vi "TGA_Main.vi"() -> ()   [LabVIEW 2016]
doc: "TGA Data Logger\n\n19-Aug-2021 R. Gibson"
uses:
  TGA_Furnace_v230504.llb/Euro_Data_cluster.ctl
  TGA_Furnace_v230504.llb/Balance_Data_cluster.ctl
  TGA_Furnace_v230504.llb/Eurotherm_3504_FP.ctl
  TGA_Furnace_v230504.llb/Eurotherm_3200_Modbus_Writeable.ctl
  TGA_Furnace_v230504.llb/Euro_Cmd_cluster.ctl
  TGA_Furnace_v230504.llb/Adam_Data_cluster.ctl
  TGA_Furnace_v230504.llb/Balance_cmd_cluster.ctl
  TGA_Furnace_v230504.llb/LogInterval.ctl
  TGA_Furnace_v230504.llb/ChartWidth.ctl
  TGA_Furnace_v230504.llb/ADAM_models_enu.ctl
  TGA_Furnace_v230504.llb/Adam_ID_cluster.ctl
  TGA_Furnace_v230504.llb/MFC_ID_cluster.ctl
  TGA_Furnace_v230504.llb/MFCs_ID_cluster.ctl
  TGA_Furnace_v230504.llb/HW_Config_cluster.ctl
  TGA_Furnace_v230504.llb/Config_cluster.ctl
  TGA_Furnace_v230504.llb/Euro_Data_cluster2.ctl
  TGA_Furnace_v230504.llb/Euro_Cmd_cluster_2.ctl
  TGA_Furnace_v230504.llb/_array_numeric_54x22.ctl
  TGA_Furnace_v230504.llb/Purge_State_enum.ctl
panel:
  out "Elapsed Time (hh:mm:ss)":string="00:00:00" caption="Elapsed Time"
  out "Logging":bool
  out "Sample#":i32 caption="# Logged"
  in  "LogInterval":T1=1 caption="Logging Interval:" items=["1 second"=1, "2 seconds"=2, "5 seconds"=5, "10 seconds"=10, "20 seconds"=20, "30 seconds"=30, "1 minute"=60, "2 minutes"=120, "5 minutes"=300]
  in  "StopLog_btn":bool
  in  "StartLog_btn":bool caption="Logging"
  out "stopping":bool=TRUE
  in  "stop":bool
  in  "Tab Control":T2(tab)
  out "MFC com error":bool caption="MFC\ncom error"
  out "Flow_status_cluster":T3
  in  "start_red_btn":bool
  in  "stop_red_btn":bool
  in  "reset_alarm_btn":bool
  in  "Zero_Balance_btn":bool
  in  "Tare_Balance_btn":bool
  out "Units":string
  out "balance_nodata":bool caption="Balance"
  out "Balance":dbl=nan caption="Mass (-offset)" format="%.3f"
  in  "offset_btn":bool
  in  "Temp_SP_btn":bool
  out "eurotherm_nodata":bool caption="Balance"
  out "Eurotherm_3504":T4={"PV"=nan, "SP"=nan, "OP"=nan} {"OP" format="%.2f"}
  out "adam_nodata":bool caption="Balance"
  out "Sample Temperature":dbl(slide)=nan scale=500.0..1800.0
  in  "chart":bool=TRUE caption="update"
  out "Waveform Chart":cluster{"Mass":dbl, "PV":dbl, dbl}(graph)={"Mass"=nan, "PV"=nan, nan}
  out "Gas_Flows 2":cluster{"N2":dbl, "H2":dbl, "CO":dbl, "CO2":dbl}={"N2"=nan, "H2"=nan, "CO"=nan, "CO2"=nan} caption="Gas_Flows (l/min)" {"CO2" format="%.2f"; "CO" format="%.2f"; "H2" format="%.2f"; "N2" format="%.2f"}
  out "N2_Alarm_2":bool
  out "Purge_state_indicator":T5(ring)
  out "Remaining":i32=284 caption="Seconds\nRemaining"
  in  "Update Graph":enum32{"Run", "Pause"}(radio) caption="Update Graph:"
  in  "clear_graph":bool
  out "XY Graph":cluster{dbl[], dbl[]}[](graph)=[{[3763419058.1468678, 3763419058.6469655, 3763419059.146789, 3763419059.647493, 3763419060.147222, 3763419060.6469135, 3763419061.146755, 3763419061.6469765, 3763419062.147566, 3763419062.647289, 3763419063.146896, 3763419063.6474705, 3763419064.147414, 3763419064.647183, 3763419065.0177894, 3763419192.4616065, 3763419192.961169, 3763419193.460889, 3763419193.9610443, 3763419194.461545, 3763419194.961543, 3763419195.460842, 3763419195.961084, 3763419196.4610868, 3763419196.961397, 3763419197.460931, 3763419197.961339, 3763419198.4614997, 3763419198.9607635, 3763419199.4611425, 3763419199.961304, 3763419200.4615474, 3763419200.960755, 3763419201.4607697, 3763419201.960702, 3763419202.4607854, 3763419202.9606795, 3763419203.460756, 3763419203.961436, 3763419204.4613805, 3763419204.961012, 3763419205.460958, 3763419205.960548, 3763419206.460789, 3763419206.9607215, 3763419207.461002, 3763419207.9605246, 3763419208.4611497, 3763419208.961407, 3763419209.461351, 3763419209.961406, 3763419210.460696, 3763419210.960537, 3763419211.460704, 3763419211.9607377, 3763419212.461395, 3763419212.961053, 3763419213.4614058, 3763419213.960675, 3763419214.4606533, 3763419214.9608603, 3763419215.4614525, 3763419215.9606404, 3763419216.4609637, 3763419216.9607835, 3763419217.4605246, 3763419217.961069, 3763419218.4613957, 3763419218.96064, 3763419219.4604506, 3763419219.961275, 3763419220.4606957, 3763419220.96139, 3763419221.4610434, 3763419221.960963, 3763419222.460838, 3763419222.9611554, 3763419223.4610176, 3763419223.961055, 3763419224.461224, 3763419224.9612026, 3763419225.2077017], [nan, nan, nan, nan, nan, nan, nan, nan, nan, nan, nan, nan, nan, nan, nan, nan, nan, nan, nan, nan, nan, nan, nan, nan, nan, nan, nan, nan, nan, nan, nan, nan, nan, nan, nan, nan, nan, nan, nan, nan, nan, nan, nan, nan, nan, nan, nan, nan, nan, nan, nan, nan, nan, nan, nan, nan, nan, nan, nan, nan, nan, nan, nan, nan, nan, nan, nan, nan, nan, nan, nan, nan, nan, nan, nan, nan, nan, nan, nan, nan, nan, nan]}, {[3763419058.1468678, 3763419058.6469655, 3763419059.146789, 3763419059.647493, 3763419060.147222, 3763419060.6469135, 3763419061.146755, 3763419061.6469765, 3763419062.147566, 3763419062.647289, 3763419063.146896, 3763419063.6474705, 3763419064.147414, 3763419064.647183, 3763419065.0177894, 3763419192.4616065, 3763419192.961169, 3763419193.460889, 3763419193.9610443, 3763419194.461545, 3763419194.961543, 3763419195.460842, 3763419195.961084, 3763419196.4610868, 3763419196.961397, 3763419197.460931, 3763419197.961339, 3763419198.4614997, 3763419198.9607635, 3763419199.4611425, 3763419199.961304, 3763419200.4615474, 3763419200.960755, 3763419201.4607697, 3763419201.960702, 3763419202.4607854, 3763419202.9606795, 3763419203.460756, 3763419203.961436, 3763419204.4613805, 3763419204.961012, 3763419205.460958, 3763419205.960548, 3763419206.460789, 3763419206.9607215, 3763419207.461002, 3763419207.9605246, 3763419208.4611497, 3763419208.961407, 3763419209.461351, 3763419209.961406, 3763419210.460696, 3763419210.960537, 3763419211.460704, 3763419211.9607377, 3763419212.461395, 3763419212.961053, 3763419213.4614058, 3763419213.960675, 3763419214.4606533, 3763419214.9608603, 3763419215.4614525, 3763419215.9606404, 3763419216.4609637, 3763419216.9607835, 3763419217.4605246, 3763419217.961069, 3763419218.4613957, 3763419218.96064, 3763419219.4604506, 3763419219.961275, 3763419220.4606957, 3763419220.96139, 3763419221.4610434, 3763419221.960963, 3763419222.460838, 3763419222.9611554, 3763419223.4610176, 3763419223.961055, 3763419224.461224, 3763419224.9612026, 3763419225.2077017], [nan, nan, nan, nan, nan, nan, nan, nan, nan, nan, nan, nan, nan, nan, nan, nan, nan, nan, nan, nan, nan, nan, nan, nan, nan, nan, nan, nan, nan, nan, nan, nan, nan, nan, nan, nan, nan, nan, nan, nan, nan, nan, nan, nan, nan, nan, nan, nan, nan, nan, nan, nan, nan, nan, nan, nan, nan, nan, nan, nan, nan, nan, nan, nan, nan, nan, nan, nan, nan, nan, nan, nan, nan, nan, nan, nan, nan, nan, nan, nan, nan, nan]}, {[3763419058.1468678, 3763419058.6469655, 3763419059.146789, 3763419059.647493, 3763419060.147222, 3763419060.6469135, 3763419061.146755, 3763419061.6469765, 3763419062.147566, 3763419062.647289, 3763419063.146896, 3763419063.6474705, 3763419064.147414, 3763419064.647183, 3763419065.0177894, 3763419192.4616065, 3763419192.961169, 3763419193.460889, 3763419193.9610443, 3763419194.461545, 3763419194.961543, 3763419195.460842, 3763419195.961084, 3763419196.4610868, 3763419196.961397, 3763419197.460931, 3763419197.961339, 3763419198.4614997, 3763419198.9607635, 3763419199.4611425, 3763419199.961304, 3763419200.4615474, 3763419200.960755, 3763419201.4607697, 3763419201.960702, 3763419202.4607854, 3763419202.9606795, 3763419203.460756, 3763419203.961436, 3763419204.4613805, 3763419204.961012, 3763419205.460958, 3763419205.960548, 3763419206.460789, 3763419206.9607215, 3763419207.461002, 3763419207.9605246, 3763419208.4611497, 3763419208.961407, 3763419209.461351, 3763419209.961406, 3763419210.460696, 3763419210.960537, 3763419211.460704, 3763419211.9607377, 3763419212.461395, 3763419212.961053, 3763419213.4614058, 3763419213.960675, 3763419214.4606533, 3763419214.9608603, 3763419215.4614525, 3763419215.9606404, 3763419216.4609637, 3763419216.9607835, 3763419217.4605246, 3763419217.961069, 3763419218.4613957, 3763419218.96064, 3763419219.4604506, 3763419219.961275, 3763419220.4606957, 3763419220.96139, 3763419221.4610434, 3763419221.960963, 3763419222.460838, 3763419222.9611554, 3763419223.4610176, 3763419223.961055, 3763419224.461224, 3763419224.9612026, 3763419225.2077017], [nan, nan, nan, nan, nan, nan, nan, nan, nan, nan, nan, nan, nan, nan, nan, nan, nan, nan, nan, nan, nan, nan, nan, nan, nan, nan, nan, nan, nan, nan, nan, nan, nan, nan, nan, nan, nan, nan, nan, nan, nan, nan, nan, nan, nan, nan, nan, nan, nan, nan, nan, nan, nan, nan, nan, nan, nan, nan, nan, nan, nan, nan, nan, nan, nan, nan, nan, nan, nan, nan, nan, nan, nan, nan, nan, nan, nan, nan, nan, nan, nan, nan]}]
  in  "GraphWidth":T6=1 caption="Graph Width" items=["1 Minute", "5 Minutes", "10 Minutes", "30 Minutes", "1 Hour", "2 Hours"]
  out "Cluster":T7={"Balance"=nan, "Furnace"=nan, "Sample"=nan} {"Balance" format="%.3f"}
  in  "test flow":dbl[](array[numeric])
  in  "Gas_Times":cluster{"Reduction Time":i32, "Purge Time":i32}={"Reduction Time"=600, "Purge Time"=300} caption="Gas Times"
  in  "Purge Flow":dbl=10.0 min=0.0 max=20.0
  in  "reset_btn2":bool
  out "N2_Alarm":bool caption="N2 Low Flow\nAlarm"
  in  "AlarmDelay":dbl=30.0 caption="N2 Low Flow\nAlarm Delay" min=1.0 max=600.0 step=1.0
  out "Gasfile_changed":bool
  out "Actual Flow (l/min)":dbl=nan caption="Total Flow" format="%.2f"
  out "Gas_Filename":string="Default+H" caption="Gas File Name"
  in  "gasfile_open_btn":bool
  in  "gasfile_saveas_btn":bool
  in  "gasfile_save_btn":bool
  in  "Gas_Controls":T8 caption="Gas On/off\nControls"
  in  "Gas Setpoints":T9={"Flow SP (l/min)"=15.0, "F1 N2 (%)"=68.0, "F1 H2 (%)"=2.0000000000000004, "F1 CO (%)"=10.0, "F1 CO2 (%)"=20.0} {"F1 H2 (%)" min=0.0 max=100.0 step=0.1 format="%.1f"; "F1 CO2 (%)" min=0.0 max=100.0 step=0.1 format="%.1f"; "F1 CO (%)" min=0.0 max=100.0 step=0.1 format="%.1f"; "F1 N2 (%)" min=-10.0 max=100.0 format="%.1f"; "Flow SP (l/min)" min=0.0 max=30.0 format="%.1f"}
  out "Sol Valve States":bool[](array[boolean])=[FALSE, FALSE, TRUE, TRUE] caption="MFC Solenoid \nValve State"
  out "MFC Loop (ms)":u32=913
  out "MFC Update":bool[](array[boolean]) caption="Update"
  out "Actual Flows (l/min)":T10[](array[typedef])=[nan, nan, nan, nan] caption="Actual\nFlows (l/min)" format="%.2f"
  out "Read Setpoints":T10[](array[typedef]) caption="Readback\nSetpoints" format="%.2f"
  out "MFC Errors":bool[](array[boolean])=[TRUE, TRUE, TRUE, TRUE] caption="Com\nError"
  out "MFC Scan":i32=4
  out "MFC Init. Error":bool[](array[boolean])=[TRUE, TRUE, TRUE, TRUE] caption="Init. \nError"
  out "TGA_select_valve":bool caption="TGA Select\nValve status"
  out "Gas_Flows":cluster{"N2":dbl, "H2":dbl, "CO":dbl, "CO2":dbl}={"N2"=nan, "H2"=nan, "CO"=nan, "CO2"=nan} caption="Gas_Flows\n(l/min)" {"CO2" format="%.2f"; "CO" format="%.2f"; "H2" format="%.2f"; "N2" format="%.2f"}
  in  "Flow_error%":dbl=20.0 caption="Low Flowrate\nDetect Error%" format="%#_13g"
  out "N2_Flow_state":u16(ring) caption="N2 Flow state"
  out "Purge_State":T11 caption="Gas State"
  in  "Purge Setpoints":T12={"F1 N2 (%)"=99.0, "F1 H2 (%)"=1.0, "F1 CO (%)"=0.0, "F1 CO2 (%)"=0.0} caption="Post-Purge Mix" {"F1 N2 (%)" format="%.1f"; "F1 CO (%)" min=0.0 max=10.0 format="%.1f"; "F1 CO2 (%)" min=0.0 max=50.0 format="%.1f"; "F1 H2 (%)" min=0.0 max=4.0 format="%.1f"}
  out "PrePurge Time":i32=300 caption="Pre-Reduction\nPurge Time"
  out "All Gas Off":bool=TRUE
  in  "Adam_Out_FB":u16=65280
  in  "Gas_SPs_Loaded":T9={"Flow SP (l/min)"=15.0, "F1 N2 (%)"=68.0, "F1 H2 (%)"=2.0000000000000004, "F1 CO (%)"=10.0, "F1 CO2 (%)"=20.0} {"F1 H2 (%)" min=0.0 max=100.0 step=0.1 format="%.1f"; "F1 CO2 (%)" min=0.0 max=100.0 step=0.1 format="%.1f"; "F1 CO (%)" min=0.0 max=100.0 step=0.1 format="%.1f"; "F1 N2 (%)" min=-10.0 max=100.0 format="%.1f"; "Flow SP (l/min)" min=0.0 max=30.0 format="%.1f"}
  out "cancel_purge":bool
  out "lock door":bool
  out "TGA_Gas_select":bool
  out "F2_Solenoid_On":bool
  out "F1_Solenoid_On":bool
  out "Adam_Out_Error":bool=TRUE
  out "Mass-Offset":dbl=nan caption="Mass-offset" format="%.4f"
  in  "LogEndComment":bool caption="Prompt for comment at end of logging"
  in  "LogStartComment":bool caption="Prompt for comment at start of logging."
  out "Filename":string
  in  "Data directory path":path=path "C:/TGA/Data"
  out "LogDivider":i32=1
  out "Mass":dbl=nan caption="Mass (g)" format="%.4f"
  in  "Mass_offset":dbl caption="Mass Offset" format="%.4f"
  in  "GraphSizeLimit":i32=7200 caption="Graph Size Limit (s)" min=300 max=86400
  out "ClearGraph":bool
  out "Log File Path":path
  out "ChrtWidth (s)":i32=300 caption="Graph Width (s)"
  out "Balance_Data_cluster":T13={"Cmd"="Error", "Stable"=FALSE, "Mass"=nan, "Units"=""}
  out "Euro_Data_cluster":T14={"Timestamp"=3763419225.2077017, "PV"=nan, "tSP"=nan, "T_OP"=nan, "wOP"=nan, "wSP"=nan} {"Timestamp" format="%<%I:%M:%S %p>T"; "wOP" format="%.1f"; "T_OP" format="%.1f"}
  out "Adam_Data_cluster":cluster{"ComError":bool, "Adam_Data":dbl[]}={"ComError"=TRUE, "Adam_Data"=[nan, nan, nan, nan, nan, nan, nan, nan]} caption="Adam_In_Data_cluster"
  out "MFCs Listbox":i32(listbox) caption="MFC IDs list"
  out "Config_Load_Error":bool caption="Config. File Load Error  -  Default values have been used."
  out "Config_Path":path=path "C:/TGA/TGA_Main_v230404.cfg" caption="Config Path:"
  out "HW_Config_display":T15={"Balance_Port"="COM4", "Adam_Input_Port"="COM6", "Euro_Port"="COM5", "Adam_Output_Port"="COM7", "MFCs_Port"="COM10"}
  out "Slide":u8(slide)=61
  out "Author:":string="Ross Gibson"
  out "Title:":string="TGA Furnace Data Logger"
  out "App Path:":string="C:\\Users\\rkg415\\Documents\\Projects\\NIER Projects\\TGA Furnace\\Software LV2016\\V230404"
  out "LabVIEW Version:":string="2016"
  out "Date:":string="19-Apr-2023"
  out "Version:":string="v230404"
  out "Program:":string="TGA_Main.vi"
  in  "Euro_cmd_Write Cluster":T17={"Value"=FALSE, "Writeable_Registers"=5225, "Writeable_Registers 2"=5227, "Value 2"=FALSE, "Writeable_Registers 3"=5226, "Value 3"=FALSE, "d/min"=5, "Writeable_Registers 4"=5381, "Writeable_Registers 5"=5382, "deg"=200, "Writeable_Registers 6"=5412, "(m)"=20, "Writeable_Registers 7"=5445, "d/min"=5, "Writeable_Registers 8"=5446, "deg"=20, "Writeable_Registers 9"=470, "Value 4"=FALSE} {"Writeable_Registers 9" items=["Autotune"=470, "P1_Seg3_TargetSP"=5446, "P1_Seg3_RampRate"=5445, "P1_Seg2_Duration"=5412, "P1_Seg1_TargetSP"=5382, "P1_Seg1_RampRate"=5381, "P1_Reset"=5225, "P1_Hold"=5227, "P1_Run"=5226, "TG.SP"=2, "MAN.OP"=3, "PB"=6, "CTRL.A"=7, "Ti"=8, "Td"=9, "RNG.LO"=11, "RNG.HI"=12, "A1.---"=13, "A2.---"=14, "SP.SEL"=15, "D.BAND"=16, "CB.Lo"=17, "CB.HI"=18, "R2G"=19, "MTR.T"=21, "T.STAT"=23, "SP1"=24, "SP2"=25, "Rm.SP"=26, "LOC.t"=27, "MR"=28, "OP.HI"=30, "OP.LO"=31, "SAFE"=34, "SP.RAT"=35, "A1.HYS"=47, "A2.HYS"=68, "A3.HYS"=69, "A4.HYS"=71, "LD.AMP"=80, "A3.---"=81, "A4.---"=82, "LBT"=83, "F.OP"=84, "F.MOD"=85, "HYST.H"=86, "HYST.C"=88, "FILT.T"=101, "RC.FT"=102, "RC.PV"=103, "Home"=106, "SP.HI"=111, "SP.LO"=112, "ADDR"=131, "PV.Offset"=141, "C.Adj"=146, "IM"=199, "MV.IN"=202, "PV.CM"=203, "SBR"=258, "NEW.AL"=260, "LBR"=263, "A.TUNE"=270, "A-M"=273, "Ac-All"=274, "L-R"=276, "REM.%"=277, "REM.HI"=278, "REM.LO"=279, "ROP.HI"=280, "ROP.LO"=281, "A1.STS"=294, "A2.STS"=295, "A3.STS"=296, "A4.STS"=297, "LD.ALM"=304, "LK.ALM"=305, "HC.ALM"=306, "LOAD.A"=307, "HILC.A"=309, "REC.NO"=313, "StOrE"=314, "TM.CFG"=320, "TM.RES"=321, "SS.SP"=322, "SS.PWR"=323, "DWELL"=324, "THRES"=327, "End.T"=328, "SERVO"=329, "EVENT"=331, "P.CYCL"=332, "CYCLE"=33, "CTRL.H"=512, "CTRL.C"=513, "PB.UNT"=514, "Lev2.P"=515, "UNITS"=516, "Lev3.P"=517, "Conf.P"=518, "Cold"=519, "PASS.C"=520, "PASS.2"=521, "COOL.t"=524, "DEC.P"=525, "STBY.T"=530, "RAMP.UNITS"=531, "Meter"=532, "uCAL"=533, "A1.TYP"=536, "A2.TYP"=537, "A3.TYP"=538, "A4.TYP"=539, "A1.LAT"=540, "A2.LAT"=541, "A3.LAT"=542, "A4.LAT"=543, "A1.BLK"=544, "A2.BLK"=545, "A3.BLK"=546, "A4.BLK"=547, "OFS.HI"=560, "OFS.LO"=561, "PNT.HI"=562, "PNT.LO"=563, "CT.RNG"=572, "Sb.tyP"=578, "Id"=629, "GO"=769, "AO.Cal"=775, "K.LOC"=1104, "Dwel.1"=1280, "TSP.1"=1281, "RMP.1"=1282, "Dwel.2"=1283, "TSP.2"=1284, "RMP.2"=1285, "Dwel.3"=1286, "TSP.3"=1287, "RMP.3"=1288, "Dwel.4"=1289, "TSP.4"=1290, "RMP.4"=1291, "AT.R2G"=4176, "IN.TYP"=12290, "CJ.tyP"=12291, "mV.HI"=12306, "mV.LO"=12307, "L.TYPE"=12352, "L.D.IN"=12353, "L.SENS"=12361, "L.TYPE (LB)"=12368, "L.D.IN (LB)"=12369, "L.SENS (LB)"=12377, "BAUD"=12548, "PRTY"=12549, "DELAY"=12550, "RETRN"=12551, "REG.AD"=12552, "Ct.Id"=12608, "CT.SRC"=12609, "CT.LAT"=12610, "1.D.IN"=12673, "1.Func"=12675, "1.RNG"=12676, "1.SRC.A"=12678, "1.SRC.B"=12679, "1.SRC.C"=12680, "1.SRC.D"=12681, "1.SENS"=12682, "1.PLS"=12706, "2.FUNC"=12739, "2.RNG"=12740, "2.SRC.A"=12742, "2.SRC.B"=12743, "2.SRC.C"=12744, "2.SRC.D"=12745, "2.SENS"=12746, "2.PLS"=12770, "3.FUNC"=12803, "3.RNG"=12804, "3.SRC.A"=12806, "3.SRC.B"=12807, "3.SRC.C"=12808, "3.SRC.D"=12809, "3.SENS"=12810, "3.PLS"=12834, "4.FUNC"=13059, "4.SRC.A"=13062, "4.SRC.B"=13063, "4.SRC.C"=13064, "4.SRC.D"=13065, "4.SENS"=13066, "4.PLS"=13090]; "Writeable_Registers 8" items=["Autotune"=470, "P1_Seg3_TargetSP"=5446, "P1_Seg3_RampRate"=5445, "P1_Seg2_Duration"=5412, "P1_Seg1_TargetSP"=5382, "P1_Seg1_RampRate"=5381, "P1_Reset"=5225, "P1_Hold"=5227, "P1_Run"=5226, "TG.SP"=2, "MAN.OP"=3, "PB"=6, "CTRL.A"=7, "Ti"=8, "Td"=9, "RNG.LO"=11, "RNG.HI"=12, "A1.---"=13, "A2.---"=14, "SP.SEL"=15, "D.BAND"=16, "CB.Lo"=17, "CB.HI"=18, "R2G"=19, "MTR.T"=21, "T.STAT"=23, "SP1"=24, "SP2"=25, "Rm.SP"=26, "LOC.t"=27, "MR"=28, "OP.HI"=30, "OP.LO"=31, "SAFE"=34, "SP.RAT"=35, "A1.HYS"=47, "A2.HYS"=68, "A3.HYS"=69, "A4.HYS"=71, "LD.AMP"=80, "A3.---"=81, "A4.---"=82, "LBT"=83, "F.OP"=84, "F.MOD"=85, "HYST.H"=86, "HYST.C"=88, "FILT.T"=101, "RC.FT"=102, "RC.PV"=103, "Home"=106, "SP.HI"=111, "SP.LO"=112, "ADDR"=131, "PV.Offset"=141, "C.Adj"=146, "IM"=199, "MV.IN"=202, "PV.CM"=203, "SBR"=258, "NEW.AL"=260, "LBR"=263, "A.TUNE"=270, "A-M"=273, "Ac-All"=274, "L-R"=276, "REM.%"=277, "REM.HI"=278, "REM.LO"=279, "ROP.HI"=280, "ROP.LO"=281, "A1.STS"=294, "A2.STS"=295, "A3.STS"=296, "A4.STS"=297, "LD.ALM"=304, "LK.ALM"=305, "HC.ALM"=306, "LOAD.A"=307, "HILC.A"=309, "REC.NO"=313, "StOrE"=314, "TM.CFG"=320, "TM.RES"=321, "SS.SP"=322, "SS.PWR"=323, "DWELL"=324, "THRES"=327, "End.T"=328, "SERVO"=329, "EVENT"=331, "P.CYCL"=332, "CYCLE"=33, "CTRL.H"=512, "CTRL.C"=513, "PB.UNT"=514, "Lev2.P"=515, "UNITS"=516, "Lev3.P"=517, "Conf.P"=518, "Cold"=519, "PASS.C"=520, "PASS.2"=521, "COOL.t"=524, "DEC.P"=525, "STBY.T"=530, "RAMP.UNITS"=531, "Meter"=532, "uCAL"=533, "A1.TYP"=536, "A2.TYP"=537, "A3.TYP"=538, "A4.TYP"=539, "A1.LAT"=540, "A2.LAT"=541, "A3.LAT"=542, "A4.LAT"=543, "A1.BLK"=544, "A2.BLK"=545, "A3.BLK"=546, "A4.BLK"=547, "OFS.HI"=560, "OFS.LO"=561, "PNT.HI"=562, "PNT.LO"=563, "CT.RNG"=572, "Sb.tyP"=578, "Id"=629, "GO"=769, "AO.Cal"=775, "K.LOC"=1104, "Dwel.1"=1280, "TSP.1"=1281, "RMP.1"=1282, "Dwel.2"=1283, "TSP.2"=1284, "RMP.2"=1285, "Dwel.3"=1286, "TSP.3"=1287, "RMP.3"=1288, "Dwel.4"=1289, "TSP.4"=1290, "RMP.4"=1291, "AT.R2G"=4176, "IN.TYP"=12290, "CJ.tyP"=12291, "mV.HI"=12306, "mV.LO"=12307, "L.TYPE"=12352, "L.D.IN"=12353, "L.SENS"=12361, "L.TYPE (LB)"=12368, "L.D.IN (LB)"=12369, "L.SENS (LB)"=12377, "BAUD"=12548, "PRTY"=12549, "DELAY"=12550, "RETRN"=12551, "REG.AD"=12552, "Ct.Id"=12608, "CT.SRC"=12609, "CT.LAT"=12610, "1.D.IN"=12673, "1.Func"=12675, "1.RNG"=12676, "1.SRC.A"=12678, "1.SRC.B"=12679, "1.SRC.C"=12680, "1.SRC.D"=12681, "1.SENS"=12682, "1.PLS"=12706, "2.FUNC"=12739, "2.RNG"=12740, "2.SRC.A"=12742, "2.SRC.B"=12743, "2.SRC.C"=12744, "2.SRC.D"=12745, "2.SENS"=12746, "2.PLS"=12770, "3.FUNC"=12803, "3.RNG"=12804, "3.SRC.A"=12806, "3.SRC.B"=12807, "3.SRC.C"=12808, "3.SRC.D"=12809, "3.SENS"=12810, "3.PLS"=12834, "4.FUNC"=13059, "4.SRC.A"=13062, "4.SRC.B"=13063, "4.SRC.C"=13064, "4.SRC.D"=13065, "4.SENS"=13066, "4.PLS"=13090]; "Writeable_Registers 7" items=["Autotune"=470, "P1_Seg3_TargetSP"=5446, "P1_Seg3_RampRate"=5445, "P1_Seg2_Duration"=5412, "P1_Seg1_TargetSP"=5382, "P1_Seg1_RampRate"=5381, "P1_Reset"=5225, "P1_Hold"=5227, "P1_Run"=5226, "TG.SP"=2, "MAN.OP"=3, "PB"=6, "CTRL.A"=7, "Ti"=8, "Td"=9, "RNG.LO"=11, "RNG.HI"=12, "A1.---"=13, "A2.---"=14, "SP.SEL"=15, "D.BAND"=16, "CB.Lo"=17, "CB.HI"=18, "R2G"=19, "MTR.T"=21, "T.STAT"=23, "SP1"=24, "SP2"=25, "Rm.SP"=26, "LOC.t"=27, "MR"=28, "OP.HI"=30, "OP.LO"=31, "SAFE"=34, "SP.RAT"=35, "A1.HYS"=47, "A2.HYS"=68, "A3.HYS"=69, "A4.HYS"=71, "LD.AMP"=80, "A3.---"=81, "A4.---"=82, "LBT"=83, "F.OP"=84, "F.MOD"=85, "HYST.H"=86, "HYST.C"=88, "FILT.T"=101, "RC.FT"=102, "RC.PV"=103, "Home"=106, "SP.HI"=111, "SP.LO"=112, "ADDR"=131, "PV.Offset"=141, "C.Adj"=146, "IM"=199, "MV.IN"=202, "PV.CM"=203, "SBR"=258, "NEW.AL"=260, "LBR"=263, "A.TUNE"=270, "A-M"=273, "Ac-All"=274, "L-R"=276, "REM.%"=277, "REM.HI"=278, "REM.LO"=279, "ROP.HI"=280, "ROP.LO"=281, "A1.STS"=294, "A2.STS"=295, "A3.STS"=296, "A4.STS"=297, "LD.ALM"=304, "LK.ALM"=305, "HC.ALM"=306, "LOAD.A"=307, "HILC.A"=309, "REC.NO"=313, "StOrE"=314, "TM.CFG"=320, "TM.RES"=321, "SS.SP"=322, "SS.PWR"=323, "DWELL"=324, "THRES"=327, "End.T"=328, "SERVO"=329, "EVENT"=331, "P.CYCL"=332, "CYCLE"=33, "CTRL.H"=512, "CTRL.C"=513, "PB.UNT"=514, "Lev2.P"=515, "UNITS"=516, "Lev3.P"=517, "Conf.P"=518, "Cold"=519, "PASS.C"=520, "PASS.2"=521, "COOL.t"=524, "DEC.P"=525, "STBY.T"=530, "RAMP.UNITS"=531, "Meter"=532, "uCAL"=533, "A1.TYP"=536, "A2.TYP"=537, "A3.TYP"=538, "A4.TYP"=539, "A1.LAT"=540, "A2.LAT"=541, "A3.LAT"=542, "A4.LAT"=543, "A1.BLK"=544, "A2.BLK"=545, "A3.BLK"=546, "A4.BLK"=547, "OFS.HI"=560, "OFS.LO"=561, "PNT.HI"=562, "PNT.LO"=563, "CT.RNG"=572, "Sb.tyP"=578, "Id"=629, "GO"=769, "AO.Cal"=775, "K.LOC"=1104, "Dwel.1"=1280, "TSP.1"=1281, "RMP.1"=1282, "Dwel.2"=1283, "TSP.2"=1284, "RMP.2"=1285, "Dwel.3"=1286, "TSP.3"=1287, "RMP.3"=1288, "Dwel.4"=1289, "TSP.4"=1290, "RMP.4"=1291, "AT.R2G"=4176, "IN.TYP"=12290, "CJ.tyP"=12291, "mV.HI"=12306, "mV.LO"=12307, "L.TYPE"=12352, "L.D.IN"=12353, "L.SENS"=12361, "L.TYPE (LB)"=12368, "L.D.IN (LB)"=12369, "L.SENS (LB)"=12377, "BAUD"=12548, "PRTY"=12549, "DELAY"=12550, "RETRN"=12551, "REG.AD"=12552, "Ct.Id"=12608, "CT.SRC"=12609, "CT.LAT"=12610, "1.D.IN"=12673, "1.Func"=12675, "1.RNG"=12676, "1.SRC.A"=12678, "1.SRC.B"=12679, "1.SRC.C"=12680, "1.SRC.D"=12681, "1.SENS"=12682, "1.PLS"=12706, "2.FUNC"=12739, "2.RNG"=12740, "2.SRC.A"=12742, "2.SRC.B"=12743, "2.SRC.C"=12744, "2.SRC.D"=12745, "2.SENS"=12746, "2.PLS"=12770, "3.FUNC"=12803, "3.RNG"=12804, "3.SRC.A"=12806, "3.SRC.B"=12807, "3.SRC.C"=12808, "3.SRC.D"=12809, "3.SENS"=12810, "3.PLS"=12834, "4.FUNC"=13059, "4.SRC.A"=13062, "4.SRC.B"=13063, "4.SRC.C"=13064, "4.SRC.D"=13065, "4.SENS"=13066, "4.PLS"=13090]; "Writeable_Registers 6" items=["Autotune"=470, "P1_Seg3_TargetSP"=5446, "P1_Seg3_RampRate"=5445, "P1_Seg2_Duration"=5412, "P1_Seg1_TargetSP"=5382, "P1_Seg1_RampRate"=5381, "P1_Reset"=5225, "P1_Hold"=5227, "P1_Run"=5226, "TG.SP"=2, "MAN.OP"=3, "PB"=6, "CTRL.A"=7, "Ti"=8, "Td"=9, "RNG.LO"=11, "RNG.HI"=12, "A1.---"=13, "A2.---"=14, "SP.SEL"=15, "D.BAND"=16, "CB.Lo"=17, "CB.HI"=18, "R2G"=19, "MTR.T"=21, "T.STAT"=23, "SP1"=24, "SP2"=25, "Rm.SP"=26, "LOC.t"=27, "MR"=28, "OP.HI"=30, "OP.LO"=31, "SAFE"=34, "SP.RAT"=35, "A1.HYS"=47, "A2.HYS"=68, "A3.HYS"=69, "A4.HYS"=71, "LD.AMP"=80, "A3.---"=81, "A4.---"=82, "LBT"=83, "F.OP"=84, "F.MOD"=85, "HYST.H"=86, "HYST.C"=88, "FILT.T"=101, "RC.FT"=102, "RC.PV"=103, "Home"=106, "SP.HI"=111, "SP.LO"=112, "ADDR"=131, "PV.Offset"=141, "C.Adj"=146, "IM"=199, "MV.IN"=202, "PV.CM"=203, "SBR"=258, "NEW.AL"=260, "LBR"=263, "A.TUNE"=270, "A-M"=273, "Ac-All"=274, "L-R"=276, "REM.%"=277, "REM.HI"=278, "REM.LO"=279, "ROP.HI"=280, "ROP.LO"=281, "A1.STS"=294, "A2.STS"=295, "A3.STS"=296, "A4.STS"=297, "LD.ALM"=304, "LK.ALM"=305, "HC.ALM"=306, "LOAD.A"=307, "HILC.A"=309, "REC.NO"=313, "StOrE"=314, "TM.CFG"=320, "TM.RES"=321, "SS.SP"=322, "SS.PWR"=323, "DWELL"=324, "THRES"=327, "End.T"=328, "SERVO"=329, "EVENT"=331, "P.CYCL"=332, "CYCLE"=33, "CTRL.H"=512, "CTRL.C"=513, "PB.UNT"=514, "Lev2.P"=515, "UNITS"=516, "Lev3.P"=517, "Conf.P"=518, "Cold"=519, "PASS.C"=520, "PASS.2"=521, "COOL.t"=524, "DEC.P"=525, "STBY.T"=530, "RAMP.UNITS"=531, "Meter"=532, "uCAL"=533, "A1.TYP"=536, "A2.TYP"=537, "A3.TYP"=538, "A4.TYP"=539, "A1.LAT"=540, "A2.LAT"=541, "A3.LAT"=542, "A4.LAT"=543, "A1.BLK"=544, "A2.BLK"=545, "A3.BLK"=546, "A4.BLK"=547, "OFS.HI"=560, "OFS.LO"=561, "PNT.HI"=562, "PNT.LO"=563, "CT.RNG"=572, "Sb.tyP"=578, "Id"=629, "GO"=769, "AO.Cal"=775, "K.LOC"=1104, "Dwel.1"=1280, "TSP.1"=1281, "RMP.1"=1282, "Dwel.2"=1283, "TSP.2"=1284, "RMP.2"=1285, "Dwel.3"=1286, "TSP.3"=1287, "RMP.3"=1288, "Dwel.4"=1289, "TSP.4"=1290, "RMP.4"=1291, "AT.R2G"=4176, "IN.TYP"=12290, "CJ.tyP"=12291, "mV.HI"=12306, "mV.LO"=12307, "L.TYPE"=12352, "L.D.IN"=12353, "L.SENS"=12361, "L.TYPE (LB)"=12368, "L.D.IN (LB)"=12369, "L.SENS (LB)"=12377, "BAUD"=12548, "PRTY"=12549, "DELAY"=12550, "RETRN"=12551, "REG.AD"=12552, "Ct.Id"=12608, "CT.SRC"=12609, "CT.LAT"=12610, "1.D.IN"=12673, "1.Func"=12675, "1.RNG"=12676, "1.SRC.A"=12678, "1.SRC.B"=12679, "1.SRC.C"=12680, "1.SRC.D"=12681, "1.SENS"=12682, "1.PLS"=12706, "2.FUNC"=12739, "2.RNG"=12740, "2.SRC.A"=12742, "2.SRC.B"=12743, "2.SRC.C"=12744, "2.SRC.D"=12745, "2.SENS"=12746, "2.PLS"=12770, "3.FUNC"=12803, "3.RNG"=12804, "3.SRC.A"=12806, "3.SRC.B"=12807, "3.SRC.C"=12808, "3.SRC.D"=12809, "3.SENS"=12810, "3.PLS"=12834, "4.FUNC"=13059, "4.SRC.A"=13062, "4.SRC.B"=13063, "4.SRC.C"=13064, "4.SRC.D"=13065, "4.SENS"=13066, "4.PLS"=13090]; "Writeable_Registers 5" items=["Autotune"=470, "P1_Seg3_TargetSP"=5446, "P1_Seg3_RampRate"=5445, "P1_Seg2_Duration"=5412, "P1_Seg1_TargetSP"=5382, "P1_Seg1_RampRate"=5381, "P1_Reset"=5225, "P1_Hold"=5227, "P1_Run"=5226, "TG.SP"=2, "MAN.OP"=3, "PB"=6, "CTRL.A"=7, "Ti"=8, "Td"=9, "RNG.LO"=11, "RNG.HI"=12, "A1.---"=13, "A2.---"=14, "SP.SEL"=15, "D.BAND"=16, "CB.Lo"=17, "CB.HI"=18, "R2G"=19, "MTR.T"=21, "T.STAT"=23, "SP1"=24, "SP2"=25, "Rm.SP"=26, "LOC.t"=27, "MR"=28, "OP.HI"=30, "OP.LO"=31, "SAFE"=34, "SP.RAT"=35, "A1.HYS"=47, "A2.HYS"=68, "A3.HYS"=69, "A4.HYS"=71, "LD.AMP"=80, "A3.---"=81, "A4.---"=82, "LBT"=83, "F.OP"=84, "F.MOD"=85, "HYST.H"=86, "HYST.C"=88, "FILT.T"=101, "RC.FT"=102, "RC.PV"=103, "Home"=106, "SP.HI"=111, "SP.LO"=112, "ADDR"=131, "PV.Offset"=141, "C.Adj"=146, "IM"=199, "MV.IN"=202, "PV.CM"=203, "SBR"=258, "NEW.AL"=260, "LBR"=263, "A.TUNE"=270, "A-M"=273, "Ac-All"=274, "L-R"=276, "REM.%"=277, "REM.HI"=278, "REM.LO"=279, "ROP.HI"=280, "ROP.LO"=281, "A1.STS"=294, "A2.STS"=295, "A3.STS"=296, "A4.STS"=297, "LD.ALM"=304, "LK.ALM"=305, "HC.ALM"=306, "LOAD.A"=307, "HILC.A"=309, "REC.NO"=313, "StOrE"=314, "TM.CFG"=320, "TM.RES"=321, "SS.SP"=322, "SS.PWR"=323, "DWELL"=324, "THRES"=327, "End.T"=328, "SERVO"=329, "EVENT"=331, "P.CYCL"=332, "CYCLE"=33, "CTRL.H"=512, "CTRL.C"=513, "PB.UNT"=514, "Lev2.P"=515, "UNITS"=516, "Lev3.P"=517, "Conf.P"=518, "Cold"=519, "PASS.C"=520, "PASS.2"=521, "COOL.t"=524, "DEC.P"=525, "STBY.T"=530, "RAMP.UNITS"=531, "Meter"=532, "uCAL"=533, "A1.TYP"=536, "A2.TYP"=537, "A3.TYP"=538, "A4.TYP"=539, "A1.LAT"=540, "A2.LAT"=541, "A3.LAT"=542, "A4.LAT"=543, "A1.BLK"=544, "A2.BLK"=545, "A3.BLK"=546, "A4.BLK"=547, "OFS.HI"=560, "OFS.LO"=561, "PNT.HI"=562, "PNT.LO"=563, "CT.RNG"=572, "Sb.tyP"=578, "Id"=629, "GO"=769, "AO.Cal"=775, "K.LOC"=1104, "Dwel.1"=1280, "TSP.1"=1281, "RMP.1"=1282, "Dwel.2"=1283, "TSP.2"=1284, "RMP.2"=1285, "Dwel.3"=1286, "TSP.3"=1287, "RMP.3"=1288, "Dwel.4"=1289, "TSP.4"=1290, "RMP.4"=1291, "AT.R2G"=4176, "IN.TYP"=12290, "CJ.tyP"=12291, "mV.HI"=12306, "mV.LO"=12307, "L.TYPE"=12352, "L.D.IN"=12353, "L.SENS"=12361, "L.TYPE (LB)"=12368, "L.D.IN (LB)"=12369, "L.SENS (LB)"=12377, "BAUD"=12548, "PRTY"=12549, "DELAY"=12550, "RETRN"=12551, "REG.AD"=12552, "Ct.Id"=12608, "CT.SRC"=12609, "CT.LAT"=12610, "1.D.IN"=12673, "1.Func"=12675, "1.RNG"=12676, "1.SRC.A"=12678, "1.SRC.B"=12679, "1.SRC.C"=12680, "1.SRC.D"=12681, "1.SENS"=12682, "1.PLS"=12706, "2.FUNC"=12739, "2.RNG"=12740, "2.SRC.A"=12742, "2.SRC.B"=12743, "2.SRC.C"=12744, "2.SRC.D"=12745, "2.SENS"=12746, "2.PLS"=12770, "3.FUNC"=12803, "3.RNG"=12804, "3.SRC.A"=12806, "3.SRC.B"=12807, "3.SRC.C"=12808, "3.SRC.D"=12809, "3.SENS"=12810, "3.PLS"=12834, "4.FUNC"=13059, "4.SRC.A"=13062, "4.SRC.B"=13063, "4.SRC.C"=13064, "4.SRC.D"=13065, "4.SENS"=13066, "4.PLS"=13090]; "Writeable_Registers 4" items=["Autotune"=470, "P1_Seg3_TargetSP"=5446, "P1_Seg3_RampRate"=5445, "P1_Seg2_Duration"=5412, "P1_Seg1_TargetSP"=5382, "P1_Seg1_RampRate"=5381, "P1_Reset"=5225, "P1_Hold"=5227, "P1_Run"=5226, "TG.SP"=2, "MAN.OP"=3, "PB"=6, "CTRL.A"=7, "Ti"=8, "Td"=9, "RNG.LO"=11, "RNG.HI"=12, "A1.---"=13, "A2.---"=14, "SP.SEL"=15, "D.BAND"=16, "CB.Lo"=17, "CB.HI"=18, "R2G"=19, "MTR.T"=21, "T.STAT"=23, "SP1"=24, "SP2"=25, "Rm.SP"=26, "LOC.t"=27, "MR"=28, "OP.HI"=30, "OP.LO"=31, "SAFE"=34, "SP.RAT"=35, "A1.HYS"=47, "A2.HYS"=68, "A3.HYS"=69, "A4.HYS"=71, "LD.AMP"=80, "A3.---"=81, "A4.---"=82, "LBT"=83, "F.OP"=84, "F.MOD"=85, "HYST.H"=86, "HYST.C"=88, "FILT.T"=101, "RC.FT"=102, "RC.PV"=103, "Home"=106, "SP.HI"=111, "SP.LO"=112, "ADDR"=131, "PV.Offset"=141, "C.Adj"=146, "IM"=199, "MV.IN"=202, "PV.CM"=203, "SBR"=258, "NEW.AL"=260, "LBR"=263, "A.TUNE"=270, "A-M"=273, "Ac-All"=274, "L-R"=276, "REM.%"=277, "REM.HI"=278, "REM.LO"=279, "ROP.HI"=280, "ROP.LO"=281, "A1.STS"=294, "A2.STS"=295, "A3.STS"=296, "A4.STS"=297, "LD.ALM"=304, "LK.ALM"=305, "HC.ALM"=306, "LOAD.A"=307, "HILC.A"=309, "REC.NO"=313, "StOrE"=314, "TM.CFG"=320, "TM.RES"=321, "SS.SP"=322, "SS.PWR"=323, "DWELL"=324, "THRES"=327, "End.T"=328, "SERVO"=329, "EVENT"=331, "P.CYCL"=332, "CYCLE"=33, "CTRL.H"=512, "CTRL.C"=513, "PB.UNT"=514, "Lev2.P"=515, "UNITS"=516, "Lev3.P"=517, "Conf.P"=518, "Cold"=519, "PASS.C"=520, "PASS.2"=521, "COOL.t"=524, "DEC.P"=525, "STBY.T"=530, "RAMP.UNITS"=531, "Meter"=532, "uCAL"=533, "A1.TYP"=536, "A2.TYP"=537, "A3.TYP"=538, "A4.TYP"=539, "A1.LAT"=540, "A2.LAT"=541, "A3.LAT"=542, "A4.LAT"=543, "A1.BLK"=544, "A2.BLK"=545, "A3.BLK"=546, "A4.BLK"=547, "OFS.HI"=560, "OFS.LO"=561, "PNT.HI"=562, "PNT.LO"=563, "CT.RNG"=572, "Sb.tyP"=578, "Id"=629, "GO"=769, "AO.Cal"=775, "K.LOC"=1104, "Dwel.1"=1280, "TSP.1"=1281, "RMP.1"=1282, "Dwel.2"=1283, "TSP.2"=1284, "RMP.2"=1285, "Dwel.3"=1286, "TSP.3"=1287, "RMP.3"=1288, "Dwel.4"=1289, "TSP.4"=1290, "RMP.4"=1291, "AT.R2G"=4176, "IN.TYP"=12290, "CJ.tyP"=12291, "mV.HI"=12306, "mV.LO"=12307, "L.TYPE"=12352, "L.D.IN"=12353, "L.SENS"=12361, "L.TYPE (LB)"=12368, "L.D.IN (LB)"=12369, "L.SENS (LB)"=12377, "BAUD"=12548, "PRTY"=12549, "DELAY"=12550, "RETRN"=12551, "REG.AD"=12552, "Ct.Id"=12608, "CT.SRC"=12609, "CT.LAT"=12610, "1.D.IN"=12673, "1.Func"=12675, "1.RNG"=12676, "1.SRC.A"=12678, "1.SRC.B"=12679, "1.SRC.C"=12680, "1.SRC.D"=12681, "1.SENS"=12682, "1.PLS"=12706, "2.FUNC"=12739, "2.RNG"=12740, "2.SRC.A"=12742, "2.SRC.B"=12743, "2.SRC.C"=12744, "2.SRC.D"=12745, "2.SENS"=12746, "2.PLS"=12770, "3.FUNC"=12803, "3.RNG"=12804, "3.SRC.A"=12806, "3.SRC.B"=12807, "3.SRC.C"=12808, "3.SRC.D"=12809, "3.SENS"=12810, "3.PLS"=12834, "4.FUNC"=13059, "4.SRC.A"=13062, "4.SRC.B"=13063, "4.SRC.C"=13064, "4.SRC.D"=13065, "4.SENS"=13066, "4.PLS"=13090]; "Writeable_Registers 3" items=["Autotune"=470, "P1_Seg3_TargetSP"=5446, "P1_Seg3_RampRate"=5445, "P1_Seg2_Duration"=5412, "P1_Seg1_TargetSP"=5382, "P1_Seg1_RampRate"=5381, "P1_Reset"=5225, "P1_Hold"=5227, "P1_Run"=5226, "TG.SP"=2, "MAN.OP"=3, "PB"=6, "CTRL.A"=7, "Ti"=8, "Td"=9, "RNG.LO"=11, "RNG.HI"=12, "A1.---"=13, "A2.---"=14, "SP.SEL"=15, "D.BAND"=16, "CB.Lo"=17, "CB.HI"=18, "R2G"=19, "MTR.T"=21, "T.STAT"=23, "SP1"=24, "SP2"=25, "Rm.SP"=26, "LOC.t"=27, "MR"=28, "OP.HI"=30, "OP.LO"=31, "SAFE"=34, "SP.RAT"=35, "A1.HYS"=47, "A2.HYS"=68, "A3.HYS"=69, "A4.HYS"=71, "LD.AMP"=80, "A3.---"=81, "A4.---"=82, "LBT"=83, "F.OP"=84, "F.MOD"=85, "HYST.H"=86, "HYST.C"=88, "FILT.T"=101, "RC.FT"=102, "RC.PV"=103, "Home"=106, "SP.HI"=111, "SP.LO"=112, "ADDR"=131, "PV.Offset"=141, "C.Adj"=146, "IM"=199, "MV.IN"=202, "PV.CM"=203, "SBR"=258, "NEW.AL"=260, "LBR"=263, "A.TUNE"=270, "A-M"=273, "Ac-All"=274, "L-R"=276, "REM.%"=277, "REM.HI"=278, "REM.LO"=279, "ROP.HI"=280, "ROP.LO"=281, "A1.STS"=294, "A2.STS"=295, "A3.STS"=296, "A4.STS"=297, "LD.ALM"=304, "LK.ALM"=305, "HC.ALM"=306, "LOAD.A"=307, "HILC.A"=309, "REC.NO"=313, "StOrE"=314, "TM.CFG"=320, "TM.RES"=321, "SS.SP"=322, "SS.PWR"=323, "DWELL"=324, "THRES"=327, "End.T"=328, "SERVO"=329, "EVENT"=331, "P.CYCL"=332, "CYCLE"=33, "CTRL.H"=512, "CTRL.C"=513, "PB.UNT"=514, "Lev2.P"=515, "UNITS"=516, "Lev3.P"=517, "Conf.P"=518, "Cold"=519, "PASS.C"=520, "PASS.2"=521, "COOL.t"=524, "DEC.P"=525, "STBY.T"=530, "RAMP.UNITS"=531, "Meter"=532, "uCAL"=533, "A1.TYP"=536, "A2.TYP"=537, "A3.TYP"=538, "A4.TYP"=539, "A1.LAT"=540, "A2.LAT"=541, "A3.LAT"=542, "A4.LAT"=543, "A1.BLK"=544, "A2.BLK"=545, "A3.BLK"=546, "A4.BLK"=547, "OFS.HI"=560, "OFS.LO"=561, "PNT.HI"=562, "PNT.LO"=563, "CT.RNG"=572, "Sb.tyP"=578, "Id"=629, "GO"=769, "AO.Cal"=775, "K.LOC"=1104, "Dwel.1"=1280, "TSP.1"=1281, "RMP.1"=1282, "Dwel.2"=1283, "TSP.2"=1284, "RMP.2"=1285, "Dwel.3"=1286, "TSP.3"=1287, "RMP.3"=1288, "Dwel.4"=1289, "TSP.4"=1290, "RMP.4"=1291, "AT.R2G"=4176, "IN.TYP"=12290, "CJ.tyP"=12291, "mV.HI"=12306, "mV.LO"=12307, "L.TYPE"=12352, "L.D.IN"=12353, "L.SENS"=12361, "L.TYPE (LB)"=12368, "L.D.IN (LB)"=12369, "L.SENS (LB)"=12377, "BAUD"=12548, "PRTY"=12549, "DELAY"=12550, "RETRN"=12551, "REG.AD"=12552, "Ct.Id"=12608, "CT.SRC"=12609, "CT.LAT"=12610, "1.D.IN"=12673, "1.Func"=12675, "1.RNG"=12676, "1.SRC.A"=12678, "1.SRC.B"=12679, "1.SRC.C"=12680, "1.SRC.D"=12681, "1.SENS"=12682, "1.PLS"=12706, "2.FUNC"=12739, "2.RNG"=12740, "2.SRC.A"=12742, "2.SRC.B"=12743, "2.SRC.C"=12744, "2.SRC.D"=12745, "2.SENS"=12746, "2.PLS"=12770, "3.FUNC"=12803, "3.RNG"=12804, "3.SRC.A"=12806, "3.SRC.B"=12807, "3.SRC.C"=12808, "3.SRC.D"=12809, "3.SENS"=12810, "3.PLS"=12834, "4.FUNC"=13059, "4.SRC.A"=13062, "4.SRC.B"=13063, "4.SRC.C"=13064, "4.SRC.D"=13065, "4.SENS"=13066, "4.PLS"=13090]; "Writeable_Registers 2" items=["Autotune"=470, "P1_Seg3_TargetSP"=5446, "P1_Seg3_RampRate"=5445, "P1_Seg2_Duration"=5412, "P1_Seg1_TargetSP"=5382, "P1_Seg1_RampRate"=5381, "P1_Reset"=5225, "P1_Hold"=5227, "P1_Run"=5226, "TG.SP"=2, "MAN.OP"=3, "PB"=6, "CTRL.A"=7, "Ti"=8, "Td"=9, "RNG.LO"=11, "RNG.HI"=12, "A1.---"=13, "A2.---"=14, "SP.SEL"=15, "D.BAND"=16, "CB.Lo"=17, "CB.HI"=18, "R2G"=19, "MTR.T"=21, "T.STAT"=23, "SP1"=24, "SP2"=25, "Rm.SP"=26, "LOC.t"=27, "MR"=28, "OP.HI"=30, "OP.LO"=31, "SAFE"=34, "SP.RAT"=35, "A1.HYS"=47, "A2.HYS"=68, "A3.HYS"=69, "A4.HYS"=71, "LD.AMP"=80, "A3.---"=81, "A4.---"=82, "LBT"=83, "F.OP"=84, "F.MOD"=85, "HYST.H"=86, "HYST.C"=88, "FILT.T"=101, "RC.FT"=102, "RC.PV"=103, "Home"=106, "SP.HI"=111, "SP.LO"=112, "ADDR"=131, "PV.Offset"=141, "C.Adj"=146, "IM"=199, "MV.IN"=202, "PV.CM"=203, "SBR"=258, "NEW.AL"=260, "LBR"=263, "A.TUNE"=270, "A-M"=273, "Ac-All"=274, "L-R"=276, "REM.%"=277, "REM.HI"=278, "REM.LO"=279, "ROP.HI"=280, "ROP.LO"=281, "A1.STS"=294, "A2.STS"=295, "A3.STS"=296, "A4.STS"=297, "LD.ALM"=304, "LK.ALM"=305, "HC.ALM"=306, "LOAD.A"=307, "HILC.A"=309, "REC.NO"=313, "StOrE"=314, "TM.CFG"=320, "TM.RES"=321, "SS.SP"=322, "SS.PWR"=323, "DWELL"=324, "THRES"=327, "End.T"=328, "SERVO"=329, "EVENT"=331, "P.CYCL"=332, "CYCLE"=33, "CTRL.H"=512, "CTRL.C"=513, "PB.UNT"=514, "Lev2.P"=515, "UNITS"=516, "Lev3.P"=517, "Conf.P"=518, "Cold"=519, "PASS.C"=520, "PASS.2"=521, "COOL.t"=524, "DEC.P"=525, "STBY.T"=530, "RAMP.UNITS"=531, "Meter"=532, "uCAL"=533, "A1.TYP"=536, "A2.TYP"=537, "A3.TYP"=538, "A4.TYP"=539, "A1.LAT"=540, "A2.LAT"=541, "A3.LAT"=542, "A4.LAT"=543, "A1.BLK"=544, "A2.BLK"=545, "A3.BLK"=546, "A4.BLK"=547, "OFS.HI"=560, "OFS.LO"=561, "PNT.HI"=562, "PNT.LO"=563, "CT.RNG"=572, "Sb.tyP"=578, "Id"=629, "GO"=769, "AO.Cal"=775, "K.LOC"=1104, "Dwel.1"=1280, "TSP.1"=1281, "RMP.1"=1282, "Dwel.2"=1283, "TSP.2"=1284, "RMP.2"=1285, "Dwel.3"=1286, "TSP.3"=1287, "RMP.3"=1288, "Dwel.4"=1289, "TSP.4"=1290, "RMP.4"=1291, "AT.R2G"=4176, "IN.TYP"=12290, "CJ.tyP"=12291, "mV.HI"=12306, "mV.LO"=12307, "L.TYPE"=12352, "L.D.IN"=12353, "L.SENS"=12361, "L.TYPE (LB)"=12368, "L.D.IN (LB)"=12369, "L.SENS (LB)"=12377, "BAUD"=12548, "PRTY"=12549, "DELAY"=12550, "RETRN"=12551, "REG.AD"=12552, "Ct.Id"=12608, "CT.SRC"=12609, "CT.LAT"=12610, "1.D.IN"=12673, "1.Func"=12675, "1.RNG"=12676, "1.SRC.A"=12678, "1.SRC.B"=12679, "1.SRC.C"=12680, "1.SRC.D"=12681, "1.SENS"=12682, "1.PLS"=12706, "2.FUNC"=12739, "2.RNG"=12740, "2.SRC.A"=12742, "2.SRC.B"=12743, "2.SRC.C"=12744, "2.SRC.D"=12745, "2.SENS"=12746, "2.PLS"=12770, "3.FUNC"=12803, "3.RNG"=12804, "3.SRC.A"=12806, "3.SRC.B"=12807, "3.SRC.C"=12808, "3.SRC.D"=12809, "3.SENS"=12810, "3.PLS"=12834, "4.FUNC"=13059, "4.SRC.A"=13062, "4.SRC.B"=13063, "4.SRC.C"=13064, "4.SRC.D"=13065, "4.SENS"=13066, "4.PLS"=13090]; "Writeable_Registers" items=["Autotune"=470, "P1_Seg3_TargetSP"=5446, "P1_Seg3_RampRate"=5445, "P1_Seg2_Duration"=5412, "P1_Seg1_TargetSP"=5382, "P1_Seg1_RampRate"=5381, "P1_Reset"=5225, "P1_Hold"=5227, "P1_Run"=5226, "TG.SP"=2, "MAN.OP"=3, "PB"=6, "CTRL.A"=7, "Ti"=8, "Td"=9, "RNG.LO"=11, "RNG.HI"=12, "A1.---"=13, "A2.---"=14, "SP.SEL"=15, "D.BAND"=16, "CB.Lo"=17, "CB.HI"=18, "R2G"=19, "MTR.T"=21, "T.STAT"=23, "SP1"=24, "SP2"=25, "Rm.SP"=26, "LOC.t"=27, "MR"=28, "OP.HI"=30, "OP.LO"=31, "SAFE"=34, "SP.RAT"=35, "A1.HYS"=47, "A2.HYS"=68, "A3.HYS"=69, "A4.HYS"=71, "LD.AMP"=80, "A3.---"=81, "A4.---"=82, "LBT"=83, "F.OP"=84, "F.MOD"=85, "HYST.H"=86, "HYST.C"=88, "FILT.T"=101, "RC.FT"=102, "RC.PV"=103, "Home"=106, "SP.HI"=111, "SP.LO"=112, "ADDR"=131, "PV.Offset"=141, "C.Adj"=146, "IM"=199, "MV.IN"=202, "PV.CM"=203, "SBR"=258, "NEW.AL"=260, "LBR"=263, "A.TUNE"=270, "A-M"=273, "Ac-All"=274, "L-R"=276, "REM.%"=277, "REM.HI"=278, "REM.LO"=279, "ROP.HI"=280, "ROP.LO"=281, "A1.STS"=294, "A2.STS"=295, "A3.STS"=296, "A4.STS"=297, "LD.ALM"=304, "LK.ALM"=305, "HC.ALM"=306, "LOAD.A"=307, "HILC.A"=309, "REC.NO"=313, "StOrE"=314, "TM.CFG"=320, "TM.RES"=321, "SS.SP"=322, "SS.PWR"=323, "DWELL"=324, "THRES"=327, "End.T"=328, "SERVO"=329, "EVENT"=331, "P.CYCL"=332, "CYCLE"=33, "CTRL.H"=512, "CTRL.C"=513, "PB.UNT"=514, "Lev2.P"=515, "UNITS"=516, "Lev3.P"=517, "Conf.P"=518, "Cold"=519, "PASS.C"=520, "PASS.2"=521, "COOL.t"=524, "DEC.P"=525, "STBY.T"=530, "RAMP.UNITS"=531, "Meter"=532, "uCAL"=533, "A1.TYP"=536, "A2.TYP"=537, "A3.TYP"=538, "A4.TYP"=539, "A1.LAT"=540, "A2.LAT"=541, "A3.LAT"=542, "A4.LAT"=543, "A1.BLK"=544, "A2.BLK"=545, "A3.BLK"=546, "A4.BLK"=547, "OFS.HI"=560, "OFS.LO"=561, "PNT.HI"=562, "PNT.LO"=563, "CT.RNG"=572, "Sb.tyP"=578, "Id"=629, "GO"=769, "AO.Cal"=775, "K.LOC"=1104, "Dwel.1"=1280, "TSP.1"=1281, "RMP.1"=1282, "Dwel.2"=1283, "TSP.2"=1284, "RMP.2"=1285, "Dwel.3"=1286, "TSP.3"=1287, "RMP.3"=1288, "Dwel.4"=1289, "TSP.4"=1290, "RMP.4"=1291, "AT.R2G"=4176, "IN.TYP"=12290, "CJ.tyP"=12291, "mV.HI"=12306, "mV.LO"=12307, "L.TYPE"=12352, "L.D.IN"=12353, "L.SENS"=12361, "L.TYPE (LB)"=12368, "L.D.IN (LB)"=12369, "L.SENS (LB)"=12377, "BAUD"=12548, "PRTY"=12549, "DELAY"=12550, "RETRN"=12551, "REG.AD"=12552, "Ct.Id"=12608, "CT.SRC"=12609, "CT.LAT"=12610, "1.D.IN"=12673, "1.Func"=12675, "1.RNG"=12676, "1.SRC.A"=12678, "1.SRC.B"=12679, "1.SRC.C"=12680, "1.SRC.D"=12681, "1.SENS"=12682, "1.PLS"=12706, "2.FUNC"=12739, "2.RNG"=12740, "2.SRC.A"=12742, "2.SRC.B"=12743, "2.SRC.C"=12744, "2.SRC.D"=12745, "2.SENS"=12746, "2.PLS"=12770, "3.FUNC"=12803, "3.RNG"=12804, "3.SRC.A"=12806, "3.SRC.B"=12807, "3.SRC.C"=12808, "3.SRC.D"=12809, "3.SENS"=12810, "3.PLS"=12834, "4.FUNC"=13059, "4.SRC.A"=13062, "4.SRC.B"=13063, "4.SRC.C"=13064, "4.SRC.D"=13065, "4.SENS"=13066, "4.PLS"=13090]}
  out "Prog read variables":T18
  # "Ack"
  # "Mode"
  # "Eurotherm"
  # "3504"
  # "°C"
  # "no alarm"
  # "Mass Flow Controllers Status"
  # "N2"
  # "H2"
  # "CO"
  # "CO2"
  # "s"
  # "s"
  # "l/min"
  # "s"
  # "open"
  # "s"
  # "Adam_Out_Status"
  # "Data Logging Settings"
  # "Centre for Ironmaking Materials Research\nNewcastle Institute for Energy and Resources (NIER)"
  # "1 = Reset\n2 = Run\n4 = Hold"
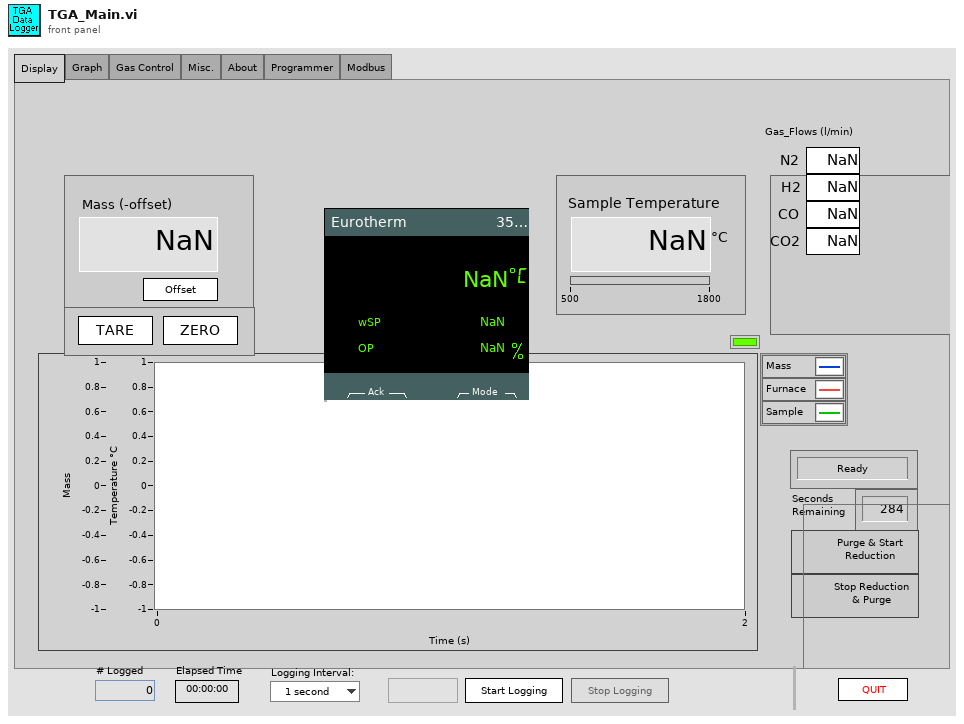
[diagram p1: front panel]
types:
  T1 = typedef "LogInterval.ctl" = u16
  T2 = enum32{"Display", "Graph", "Gas Control", "Misc.", "About", "Programmer", "Modbus"}
  T3 = cluster{"N2_Flow_state":u16, "H2_Flow_state":u16, "CO_Flow_state":u16, "CO2_Flow_state":u16}
  T4 = typedef "Eurotherm_3504_FP.ctl" = cluster{"PV":dbl, "SP":dbl, "OP":dbl}
  T5 = enum16{"Ready", "StartPrePurge", "PrePurge", "StartReduction", "Reduction", "StartPostPurge", "PostPurge"}
  T6 = typedef "ChartWidth.ctl" = u16
  T7 = cluster{"Balance":dbl, "Furnace":dbl, "Sample":dbl}
  T8 = cluster{"N2 On":bool, "H2 On":bool, "CO On":bool, "CO2 On":bool}
  T9 = cluster{"Flow SP (l/min)":dbl, "F1 N2 (%)":dbl, "F1 H2 (%)":dbl, "F1 CO (%)":dbl, "F1 CO2 (%)":dbl}
  T10 = typedef "_array_numeric_54x22.ctl" = dbl
  T11 = typedef "Purge_State_enum.ctl" = enum16{"Ready", "StartPrePurge", "PrePurge", "StartReduction", "Reduction", "StartPostPurge", "PostPurge"}
  T12 = cluster{"F1 N2 (%)":dbl, "F1 H2 (%)":dbl, "F1 CO (%)":dbl, "F1 CO2 (%)":dbl}
  T13 = typedef "Balance_Data_cluster.ctl" = cluster{"Cmd":string, "Stable":bool, "Mass":dbl, "Units":string}
  T14 = cluster{"Timestamp":dbl, "PV":dbl, "tSP":dbl, "T_OP":dbl, "wOP":dbl, "wSP":dbl}
  T15 = cluster{"Balance_Port":refnum<visa-resource-name>, "Adam_Input_Port":refnum<visa-resource-name>, "Euro_Port":refnum<visa-resource-name>, "Adam_Output_Port":refnum<visa-resource-name>, "MFCs_Port":refnum<visa-resource-name>}
  T16 = typedef "Eurotherm_3200_Modbus_Writeable.ctl" = u16
  T17 = cluster{"Value":bool, "Writeable_Registers":T16, "Writeable_Registers 2":T16, "Value 2":bool, "Writeable_Registers 3":T16, "Value 3":bool, "d/min":u16, "Writeable_Registers 4":T16, "Writeable_Registers 5":T16, "deg":u16, "Writeable_Registers 6":T16, "(m)":u16, "Writeable_Registers 7":T16, "d/min":u16, "Writeable_Registers 8":T16, "deg":u16, "Writeable_Registers 9":T16, "Value 4":bool}
  T18 = cluster{"Current Prog Time Left":u16, "Current Prog Status":u16, "Current Prog Segment":u16, "Current Prog Number":u16, "Current Prog Seg Type":u16, "Current Prog Seg Time Left":u16, "Pb":u16, "ti":u16, "td":u16}
  T19 = enum32{"Display", "Graph", "Gas Control", "Misc.", "About"}
  T20 = enum32{"Invalid", "Standard", "Closed", "Hidden", "Minimized", "Maximized"}
  T21 = typedef "Config_cluster.ctl" = cluster{"ConfigFile path":path, "Data directory path":path, "LogInterval":T1, "LogStartComment":bool, "LogEndComment":bool, "GraphWidth":T6, "GraphSizeLimit":u16, "HW_Config_cluster":T22, "TGA Gas File":string, "Gas_SPs":cluster{"Flow SP":dbl, "N2 (%)":dbl, "H2 (%)":dbl, "CO (%)":dbl, "CO2 (%)":dbl}, "AlarmDelay":dbl, "Flow_error%":dbl, "Purge Flow":dbl, "Gas_Times":cluster{"PrePurge Time":dbl, "Reduction Time":dbl, "Purge Time":dbl}, "Purge Setpoints":cluster{"F1 N2 (%)":dbl, "F1 H2 (%)":dbl, "F1 CO (%)":dbl, "F1 CO2 (%)":dbl}}
  T22 = typedef "HW_Config_cluster.ctl" = cluster{"Balance_Port":refnum<visa-resource-name>, "Adam_In_ID":T23, "Euro_Port":refnum<visa-resource-name>, "Euro_Address":u8, "Adam_Out_ID":T23, "MFCs_Port":refnum<visa-resource-name>, "MFC Device IDs":T25}
  T23 = typedef "Adam_ID_cluster.ctl" = cluster{"Serial Port":refnum<visa-resource-name>, "Model":T24, "Address":u8, "Slot":u8}
  T24 = typedef "ADAM_models_enu.ctl" = enum16{"4011", "4012", "4013", "4015", "4015T", "4016", "4017", "4017+", "4018", "4018+", "4019+", "4019M", "4021", "4024", "4050", "4051", "4052", "4053", "4055", "4056S", "4056SO", "4060", "4068", "4069", "5000", "5017", "5018", "5024", "5051"}
  T25 = typedef "MFCs_ID_cluster.ctl" = cluster{"F1N2 MFC Device ID":T26, "F1H2 MFC Device ID":T26, "F1CO MFC Device ID":T26, "F1CO2 MFC Device ID":T26}
  T26 = typedef "MFC_ID_cluster.ctl" = cluster{"MFC Device ID":u32, "Type":u8}
  T27 = enum8{"Enabled", "Disabled", "Disabled and Grayed Out"}
  T28 = typedef "Euro_Cmd_cluster_2.ctl" = cluster{"Register":T16, "Value":bool, "Value 2":bool, "Register 2":T16, "Value 3":bool, "Register 3":T16, "Value 4":dbl, "Register 4":T16, "Value 5":dbl, "Register 5":T16, "Value 6":dbl, "Register 6":T16, "Value 7":dbl, "Register 7":T16, "Value 8":dbl, "Register 8":T16, "Value 9":dbl, "Register 9":T16}
  T29 = typedef "Euro_Data_cluster2.ctl" = cluster{dbl, dbl, dbl, dbl, dbl, dbl, dbl, dbl, dbl}
  T30 = typedef "Balance_cmd_cluster.ctl" = cluster{"cmd":enum16{"nop", "Tare", "Zero", "Lock", "Unlock", "AutoZero", "SetFilter", "Login", "Logout"}, "Value":i8}
  T31 = typedef "Adam_Data_cluster.ctl" = cluster{"ComError":bool, "Adam_Data":dbl[]}
  T32 = typedef "Euro_Cmd_cluster.ctl" = cluster{"Register":T16, "Value":dbl}
  T33 = typedef "Euro_Data_cluster.ctl" = cluster{"Timestamp":dbl, "PV":dbl, "tSP":dbl, "T_OP":dbl, "wOP":dbl, "wSP":dbl}
  T34 = cluster{"Flow SP":dbl, "N2 (%)":dbl, "H2 (%)":dbl, "CO (%)":dbl, "CO2 (%)":dbl}
  T35 = cluster{"Flow SP (l/min)":bool, "F1 N2 (%)":bool, "F1 H2 (%)":bool, "F1 CO (%)":bool, "F1 CO2 (%)":bool}
  T36 = cluster{"[0]":dbl, "[1]":dbl, "[2]":dbl, "[3]":dbl}
  T37 = cluster{"[0]":bool, "[1]":bool, "[2]":bool, "[3]":bool}
  T38 = cluster{"F1 N2 (%)":bool, "F1 H2 (%)":bool, "F1 CO (%)":bool, "F1 CO2 (%)":bool}
  T39 = typedef "LVPoint32TypeDef.ctl" = cluster{"Horizontal":i32, "Vertical":i32}
  T40 = typedef "LVRectTypeDef.ctl" = cluster{"Left":i16, "Top":i16, "Right":i16, "Bottom":i16}
  T41 = cluster{"[0]":enum16{"Off", "Ok", "Low"}, "[1]":enum16{"Off", "Ok", "Low"}, "[2]":enum16{"Off", "Ok", "Low"}, "[3]":enum16{"Off", "Ok", "Low"}}
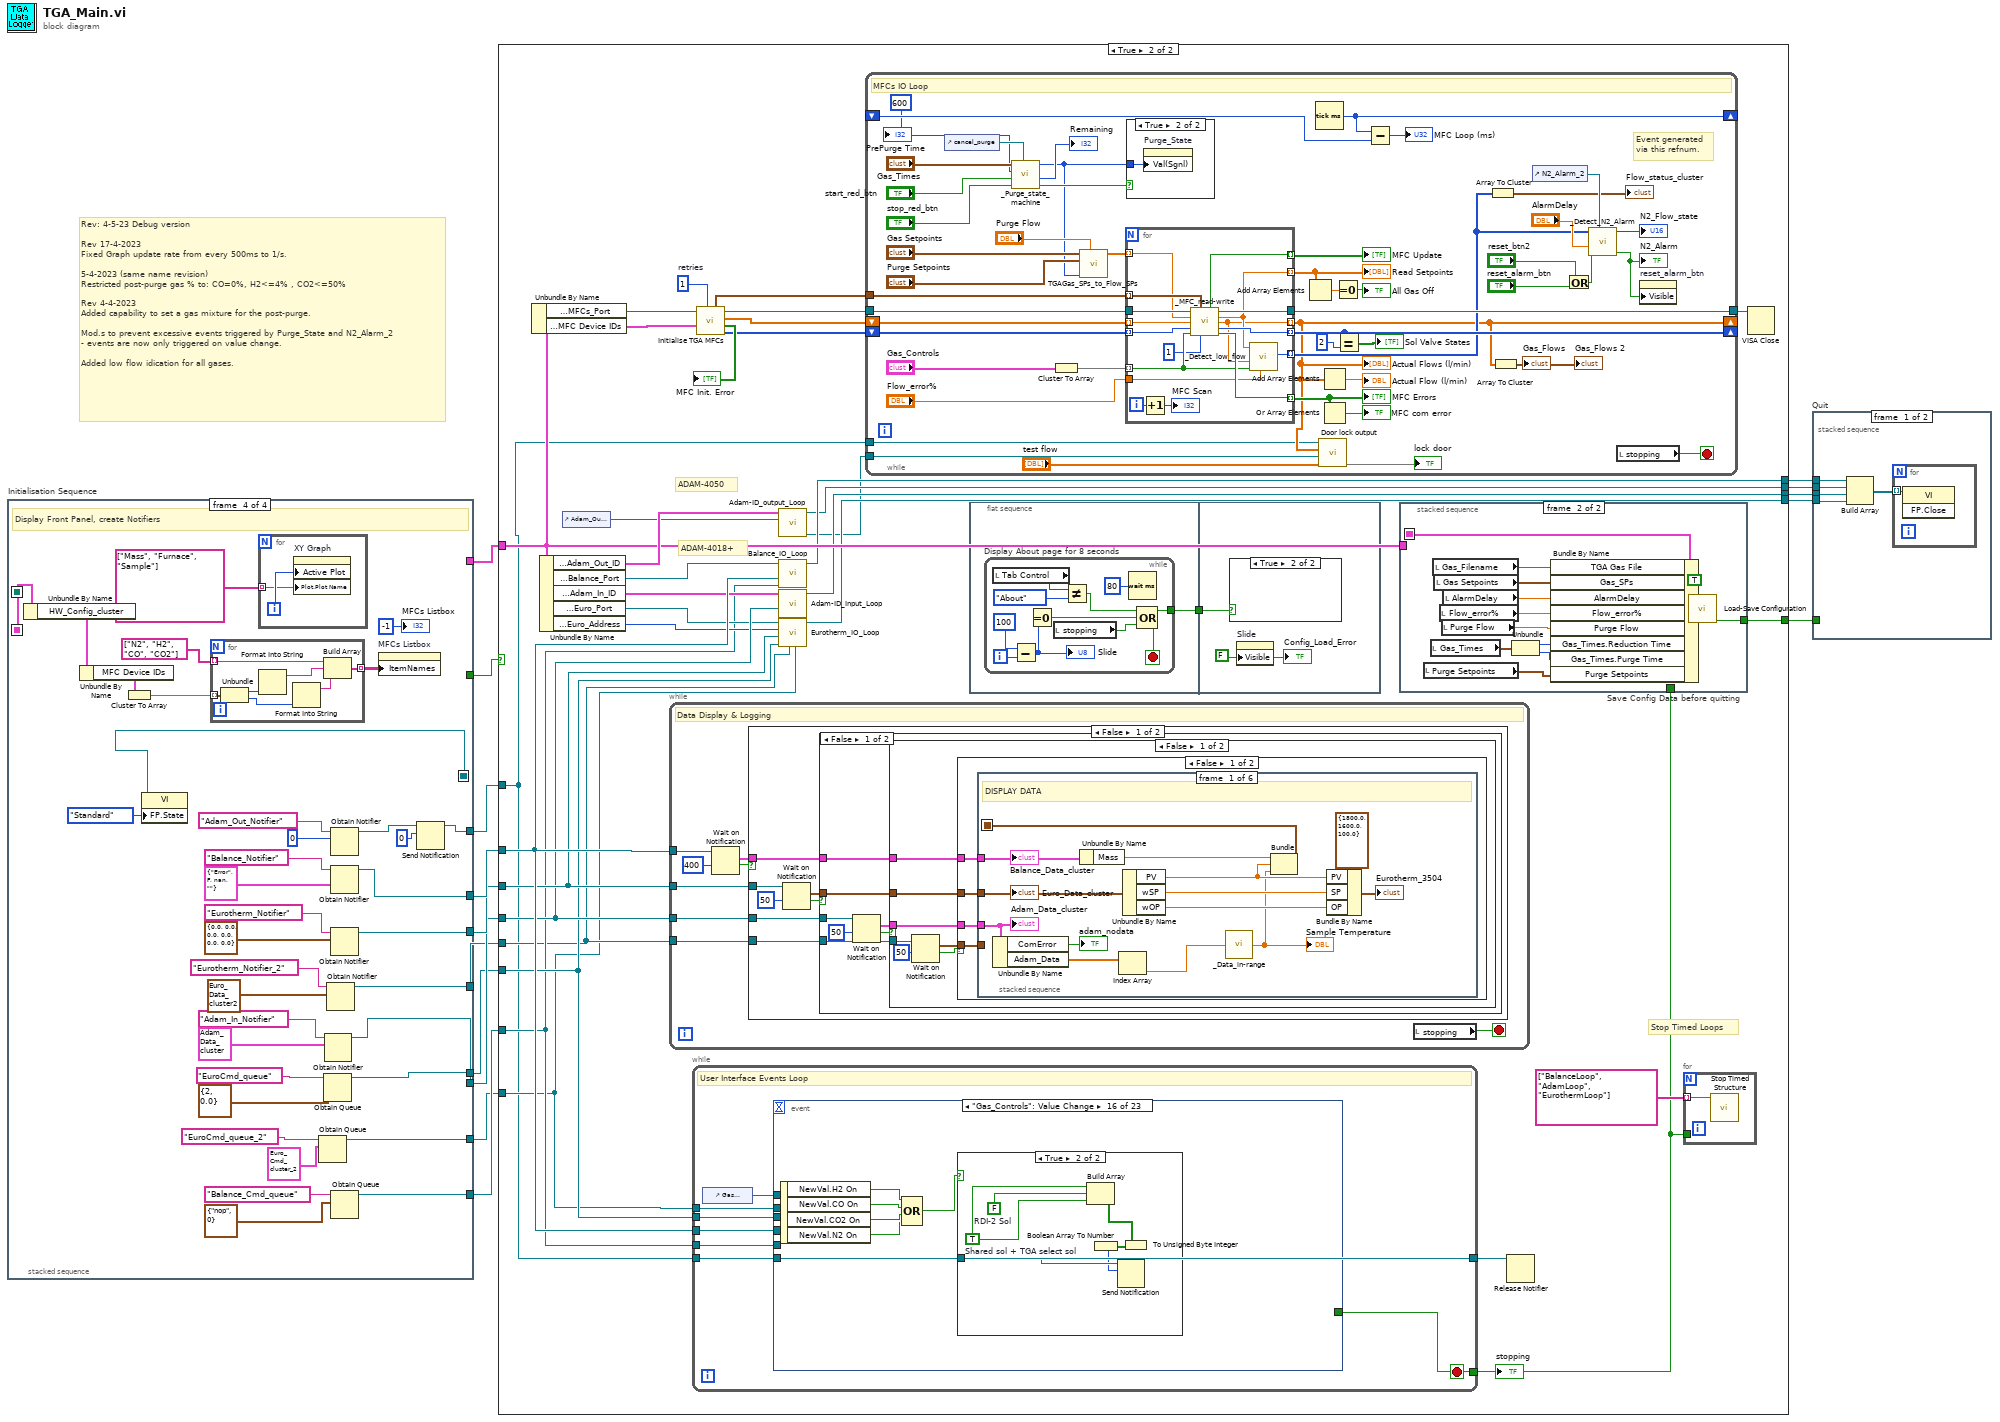
[diagram p0: block diagram]
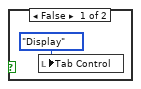
[diagram p4: hidden frame]
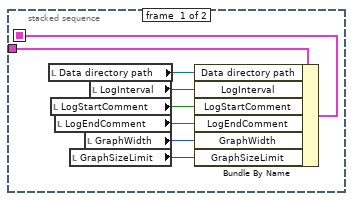
[diagram p5: hidden frame]
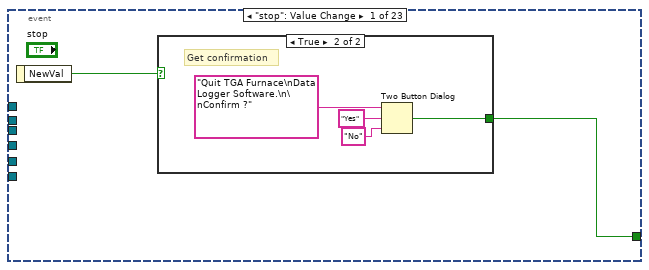
[diagram p6: hidden frame]
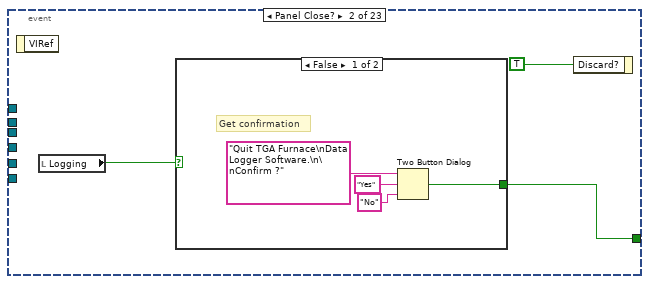
[diagram p8: hidden frame]
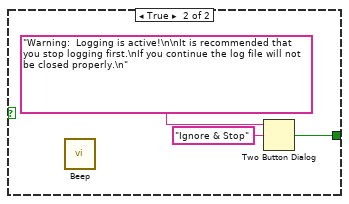
[diagram p9: hidden frame]
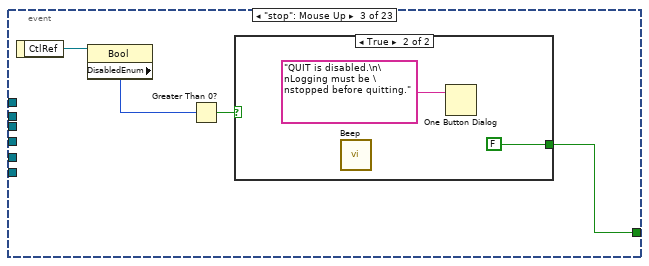
[diagram p10: hidden frame]
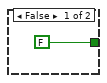
[diagram p11: hidden frame]
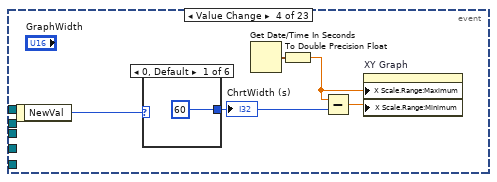
[diagram p12: hidden frame]
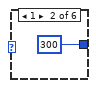
[diagram p13: hidden frame]
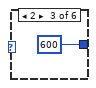
[diagram p14: hidden frame]
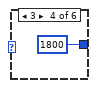
[diagram p15: hidden frame]
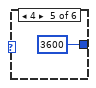
[diagram p16: hidden frame]
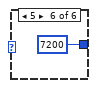
[diagram p17: hidden frame]
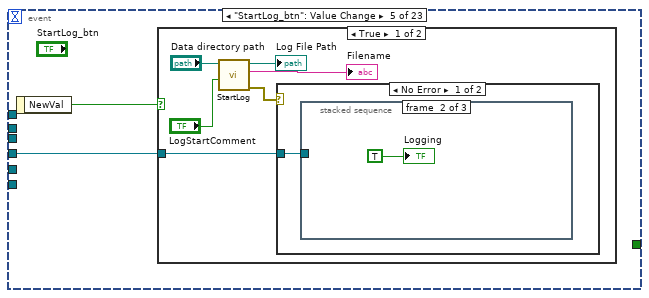
[diagram p18: hidden frame]
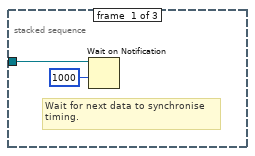
[diagram p19: hidden frame]
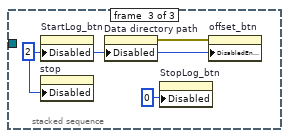
[diagram p20: hidden frame]
diagram:
  # "Rev: 4-5-23 Debug version\n\nRev 17-4-2023\nFixed Graph update rate from every 500ms to 1/s.\n\n5-4-2023 (same name revision)\nRestricted post-purge gas % to: CO=0%, H2<=4% , CO2<=50%\n\nRev 4-4-2023\nAdded capability to set a gas mixture for the post-purge.\n\nMod.s to prevent excessive events triggered by Purge_State and N2_Alarm_2 \n- events are now only triggered on value change.\n\nAdded low flow idication for all gases."
  n1 = stacked-sequence "Initialisation Sequence" {
    seq-local: [w18 _ _ _] -> [_ w39 w49 _]
    seq-local: [_ w38 _ _] -> [_ _ w48 w80]
    seq-local: [w21 _ _ _] -> [_ _ _ w96]
    tunnel: [_ _ w67 _] -> w10
    tunnel: [_ _ w68 _] -> w15
    tunnel: [_ _ _ w98] -> w13
    tunnel: [_ _ _ w99] -> w12
    tunnel: [_ _ _ w97] -> w11
    tunnel: [_ _ _ w93] -> w9
    tunnel: [_ _ _ w89] -> w8
    tunnel: [_ _ _ w85] -> w7
    tunnel: [_ _ _ w75] -> w2
    tunnel: [_ _ _ w72] -> w1
    frame #0 {
      w23 = path "C:/Users/Welcome29/Documents/GitHub/N103-TGA"  # Config_Directory
      w19 = "v240408" ("Version:")
      # "Hide Front Panel & Get/Create Paths"
      n2 = property class="VI"("FP.State"=T20."Hidden" ("Front Panel Window:State")) -> (reference out=w21:refnum<vi>)  [unwired: 2 in, 1 out]
      n3 = Current VI's Path() -> (path=w25:path)
      n4 = call <vilib>:"Application Directory.vi"() -> ("Application Directory"=w17:path)
      n5 = call "_Build_Config_Path.vi"("Version:"=w19, "Config_Directory"=w23, "Vi_path"=w25) -> ("Vi name"=→"Program:":string, "Config_Path"=w18:path)  [unwired: 6 in, 1 out]
      "Config_Path" <- w18
      n6 = Path To String(path=w17) -> (string=→"App Path:":string)
      n7 = local write "Tab Control"(T19."About" ("Tab Control")) -> ()
      "Version:" <- w19
      "LabVIEW Version:" <- "2016" ("LavVIEW Version:")
      "Date:" <- "8-April-2024" ("Date:")
      "Title:" <- "TGA Furnace Data Logger" ("Title:")
      "Author:" <- "Ross Gibson" ("Author:")
    }
    frame #1 {
      w36 = T27."Enabled" ("Disabled")
      # "Load Settings, initialise Disable property nodes"
      n8 = property on="LogInterval" class="Ring (strict)"("Disabled"=w36) -> ()  [unwired: 2 in, 2 out]
      n9 = property on="stop" class="Bool"("Disabled"=w36) -> ()  [unwired: 2 in, 2 out]
      n10 = local write "Gas_Controls"(T8 {"N2 On"=FALSE, "H2 On"=FALSE, "CO On"=FALSE, "CO2 On"=FALSE} ("Gas_Controls")) -> ()
      n11 = local write "Elapsed Time (hh:mm:ss)"("00:00:00" ("Elapsed Time (hh:mm:ss)")) -> ()
      n12 = local write "Mass_offset"(0.0 ("Mass_offset")) -> ()
      n13 = local write "Log File Path"(path "" ("Log File Path")) -> ()
      n14 = call "Load-Save Configuration.vi"("Config Cluster"=T21 {"ConfigFile path"=path "C:/TGA", "Data directory path"=path "C:/TGA/Data", "LogInterval"=1, "LogStartComment"=FALSE, "LogEndComment"=FALSE, "GraphWidth"=1, "GraphSizeLimit"=7200, "HW_Config_cluster"={"Balance_Port"="COM4", "Adam_In_ID"={"Serial Port"="COM6", "Model"=enum."4018", "Address"=1, "Slot"=0}, "Euro_Port"="COM5", "Euro_Address"=1, "Adam_Out_ID"={"Serial Port"="COM7", "Model"=enum."4050", "Address"=1, "Slot"=0}, "MFCs_Port"="COM10", "MFC Device IDs"={"F1N2 MFC Device ID"={"MFC Device ID"=751101, "Type"=50}, "F1H2 MFC Device ID"={"MFC Device ID"=98201001, "Type"=100}, "F1CO MFC Device ID"={"MFC Device ID"=751202, "Type"=50}, "F1CO2 MFC Device ID"={"MFC Device ID"=98202001, "Type"=100}}}, "TGA Gas File"="Default", "Gas_SPs"={"Flow SP"=15.0, "N2 (%)"=70.0, "H2 (%)"=0.0, "CO (%)"=10.0, "CO2 (%)"=20.0}, "AlarmDelay"=30.0, "Flow_error%"=20.0, "Purge Flow"=10.0, "Gas_Times"={"PrePurge Time"=300.0, "Reduction Time"=600.0, "Purge Time"=300.0}, "Purge Setpoints"={"F1 N2 (%)"=100.0, "F1 H2 (%)"=0.0, "F1 CO (%)"=0.0, "F1 CO2 (%)"=0.0}}, "ConfigFile path (Not A Path)"=w39) -> ("Error"=w37:bool, "Config Cluster out"=w38:T21)  [unwired: 6 in]
      n15 = property on="StartLog_btn" class="Bool"("Disabled"=w36) -> ()  [unwired: 2 in, 2 out]
      n16 = property on="StopLog_btn" class="Bool"("Disabled"=T27."Disabled and Grayed Out") -> ()  [unwired: 2 in, 2 out]
      n17 = property on="offset_btn" class="Bool"("DisabledEnum"=w36) -> ()  [unwired: 2 in, 2 out]
      n18 = property on="Config_Load_Error" class="Bool (strict)"("Visible"=w37, "Value"=w37) -> ()  [unwired: 2 in, 2 out]
    }
    frame #2 {
      w45 = FALSE ("stopping")
      # "continue ?"
      # "Find Hardware, initialise variables"
      n19 = Unbundle By Name(w48) -> ("Data directory path"=w66:path, "LogInterval"=w62:T1, "LogStartComment"=w59:bool, "LogEndComment"=w58:bool, "GraphSizeLimit"=w60:u16, "GraphWidth"=w61:T6, "TGA Gas File"=w54:string, "Gas_SPs"=w55:T34, "AlarmDelay"=w51:dbl, "Flow_error%"=w50:dbl, "Purge Flow"=w46:dbl, "Gas_Times.Reduction Time"=w41:dbl, "Gas_Times.Purge Time"=w40:dbl, "Purge Setpoints"=w43:T12)
      n20 = Unbundle By Name(w48) -> ("HW_Config_cluster"=w69:T22)
      n21 = Bundle By Name(cluster=w48, "ConfigFile path"=w49) -> (w47:T21)
      n22 = control-ref of="Gas_SPs_Loaded"() -> (w53:refnum<vi>)
      n23 = call "Find_TGA_DAQ_Hardware.vi"("HW_Config_cluster"=w69) -> ("Abort"=w70:bool, "HW_Ports_cluster"=→"HW_Config_display":T15, "HW_Config_cluster out"=w44:T22)  [unwired: 4 in, 2 out]
      n24 = local write "Slide"(u8 0 ("Slide")) -> ()
      n25 = call "_Load-Save_Gas_File.vi"("No_dialog"=TRUE, "Gas_Setpoints_ref"=w53, "Gas_Filename"=w54) -> ()  [unwired: 5 in, 4 out]
      n26 = Index Array(array=i32[] [60, 300, 600, 1800, 3600, 7200], index=w61) -> (element=w65:i32)
      n27 = Bundle("Reduction Time"=w41, "Purge Time"=w40) -> (w42:cluster{"Reduction Time":dbl, "Purge Time":dbl})  [unwired: 1 in]
      n28 = To Long Integer(number=w62) -> (32bit integer=w63:i32)
      n29 = local write "ChrtWidth (s)"(w65) -> ()
      n30 = Not(x=w70) -> (.not. x?=w67:bool)
      n31 = Bundle By Name(cluster=w47, "HW_Config_cluster"=w44) -> (w68:T21)
      n32 = local write "stopping"(w45) -> ()
      n33 = local write "Logging"(w45) -> ()
      n34 = local write "Gasfile_changed"(w45) -> ()
      n35 = local write "Purge Setpoints"(w43) -> ()
      n36 = local write "LogDivider"(w63) -> ()
      n37 = local write "Data directory path"(w66) -> ()
      n38 = local write "LogInterval"(w62) -> ()
      n39 = local write "LogStartComment"(w59) -> ()
      n40 = local write "LogEndComment"(w58) -> ()
      n41 = local write "GraphSizeLimit"(w60) -> ()
      n42 = local write "GraphWidth"(w61) -> ()
      n43 = local write "Gas_Filename"(w54) -> ()
      n44 = local write "Gas Setpoints"(w55) -> ()
      n45 = local write "AlarmDelay"(w51) -> ()
      n46 = local write "Flow_error%"(w50) -> ()
      n47 = local write "Purge Flow"(w46) -> ()
      n48 = local write "Gas_Times"(w42) -> ()
      n49 = local write "N2_Alarm_2"(w45) -> ()
      n50 = property on="Slide" class="Slide (strict)"("Visible"=w67) -> ()  [unwired: 2 in, 2 out]
    }
    frame #3 {
      # "Display Front Panel, create Notifiers"
      n51 = Unbundle By Name(w80) -> ("HW_Config_cluster"=w79:T22)
      n52 = Unbundle By Name(w79) -> ("MFC Device IDs"=w83:T25)
      n53 = Cluster To Array(cluster=w83) -> (array=w82:T26[])
      n54 = property class="VI"(reference=w96, "FP.State"=T20."Standard" ("Front Panel Window:State")) -> ()  [unwired: 1 in, 2 out]
      n55 = for {
        tunnel: w82 -> [w113] mode=indexing
        tunnel: string[] ["N2", "H2", "CO", "CO2"] -> [w111] mode=indexing
        tunnel: [w107] -> w78 mode=indexing
        n56 = Unbundle(w113) -> ("MFC Device ID"=w112:u32, "Type"=w109:u8)
        n57 = Format Into String(w112) -> (resulting string=w110:string)  [unwired: 3 in, 1 out]
        n58 = Format Into String(w109) -> (resulting string=w108:string)  [unwired: 3 in, 1 out]
        n59 = Build Array(w111, w110, w108) -> (w107:string[])
      }
      n60 = for {
        tunnel: string[] ["Mass", "Furnace", "Sample"] -> [w114] mode=indexing
        i -> [w115]
        n61 = property on="XY Graph" class="XYGraph (strict)"("Active Plot"=w115, "Plot.Plot Name"=w114) -> ()  [unwired: 2 in, 2 out]
      }
      n62 = Obtain Queue(name (unnamed)="EuroCmd_queue_2", element data type=T28 {"Register"=5446, "Value"=FALSE, "Value 2"=FALSE, "Register 2"=5445, "Value 3"=FALSE, "Register 3"=5412, "Value 4"=0.0, "Register 4"=0, "Value 5"=0.0, "Register 5"=5382, "Value 6"=0.0, "Register 6"=5412, "Value 7"=0.0, "Register 7"=5445, "Value 8"=0.0, "Register 8"=5446, "Value 9"=0.0, "Register 9"=470} ("EuroCmd_cluster_2")) -> (queue out=w72:refnum<queue>)  [unwired: 3 in, 2 out]
      n63 = Obtain Queue(name (unnamed)="EuroCmd_queue", element data type=T32 {"Register"=2, "Value"=0.0} ("Euro_Cmd_cluster")) -> (queue out=w93:refnum<queue>)  [unwired: 3 in, 2 out]
      n64 = Obtain Notifier(name (unnamed)="Adam_In_Notifier", notification data type=T31 {"ComError"=FALSE, "Adam_Data"=[nan, nan, nan, nan, nan, nan, nan, nan]} ("Adam_Data_cluster")) -> (notifier out=w97:refnum<notifier>)  [unwired: 2 in, 2 out]
      n65 = Obtain Notifier(name (unnamed)="Eurotherm_Notifier_2", notification data type=T29 {0.0, 0.0, 0.0, 0.0, 0.0, 0.0, 0.0, 0.0, 0.0} ("Programmer Read Variables")) -> (notifier out=w75:refnum<notifier>)  [unwired: 2 in, 2 out]
      n66 = Obtain Notifier(name (unnamed)="Adam_Out_Notifier", notification data type=u8 0) -> (notifier out=w86:refnum<notifier>)  [unwired: 2 in, 2 out]
      n67 = Obtain Notifier(name (unnamed)="Balance_Notifier", notification data type=T13 {"Cmd"="Error", "Stable"=FALSE, "Mass"=nan, "Units"=""} ("Balance_Data_cluster")) -> (notifier out=w98:refnum<notifier>)  [unwired: 2 in, 2 out]
      n68 = Obtain Notifier(name (unnamed)="Eurotherm_Notifier", notification data type=T33 {"Timestamp"=0.0, "PV"=0.0, "tSP"=0.0, "T_OP"=0.0, "wOP"=0.0, "wSP"=0.0} ("Euro_Data_cluster")) -> (notifier out=w99:refnum<notifier>)  [unwired: 2 in, 2 out]
      n69 = Obtain Queue(name (unnamed)="Balance_Cmd_queue", element data type=T30 {"cmd"=enum."nop", "Value"=0}) -> (queue out=w89:refnum<queue>)  [unwired: 3 in, 2 out]
      n70 = property on="MFCs Listbox" class="MCListbox (strict)"("ItemNames"=w78) -> ()  [unwired: 2 in, 2 out]
      n71 = Send Notification(notification=u8 0, notifier=w86) -> (notifier out=w85:refnum<notifier>)  [unwired: 1 in, 1 out]
      "MFCs Listbox" <- -1 ("MFCs Listbox")
    }
  }
  n72 = case shown="True" w10 {
    selector: w10 -> [w116 _]
    tunnel: w15 -> [_ w129]
    tunnel: [w116 w150] -> w14
    tunnel: w13 -> [_ w147]
    tunnel: w12 -> [_ w146]
    tunnel: w11 -> [_ w145]
    tunnel: w9 -> [_ w139]
    tunnel: w8 -> [_ w138]
    tunnel: w7 -> [_ w118]
    tunnel: [_ w124] -> w6
    tunnel: [_ w123] -> w5
    tunnel: [_ w122] -> w4
    tunnel: [_ w121] -> w3
    tunnel: w2 -> [_ w120]
    tunnel: w1 -> [_ w119]
    frame False {
      # "Hardware not found - do nothing"
    }
    frame True {
      w125 = 1  # retries
      # "Stop Timed Loops"
      # "ADAM-4018+"
      # "ADAM-4050"
      n73 = Unbundle By Name(w129) -> ("HW_Config_cluster.MFCs_Port"=w128:refnum<visa-resource-name>, "HW_Config_cluster.MFC Device IDs"=w127:T25)
      n74 = Unbundle By Name(w129) -> ("HW_Config_cluster.Adam_Out_ID"=w137:T23, "HW_Config_cluster.Balance_Port"=w144:refnum<visa-resource-name>, "HW_Config_cluster.Adam_In_ID"=w143:T23, "HW_Config_cluster.Euro_Port"=w142:refnum<visa-resource-name>, "HW_Config_cluster.Euro_Address"=w141:u8)
      n75 = control-ref of="Adam_Out_FB"() -> (w136:refnum<vi>)
      n76 = while "Data Display & Logging" {
        tunnel: w147 -> [w488]
        tunnel: w146 -> [w484]
        tunnel: w145 -> [w483]
        tunnel: w120 -> [w481]
        stop <- w482 stop-if-true
        # "Data Display & Logging"
        n77 = Wait on Notification(notifier=w488, timeout in ms (-1)=400) -> (notification=w487:T13, timed out?=w486:bool)  [unwired: 2 in, 2 out]
        n78 = case shown="False" w486 {
          tunnel: w487 -> [w490 _]
          tunnel: w484 -> [w494 _]
          tunnel: w483 -> [w491 _]
          tunnel: w481 -> [w489 _]
          frame False {
            n79 = Wait on Notification(notifier=w494, timeout in ms (-1)=50) -> (notification=w492:T33, timed out?=w493:bool)  [unwired: 2 in, 2 out]
            n80 = case shown="False" w493 {
              tunnel: w492 -> [w497 _]
              tunnel: w491 -> [w501 _]
              tunnel: w490 -> [w498 _]
              tunnel: w489 -> [w496 _]
              frame False {
                n81 = Wait on Notification(notifier=w501, timeout in ms (-1)=50) -> (notification=w499:T31, timed out?=w500:bool)  [unwired: 2 in, 2 out]
                n82 = case shown="False" w500 {
                  tunnel: w499 -> [w508 _]
                  tunnel: w498 -> [w507 _]
                  tunnel: w497 -> [w509 _]
                  tunnel: w496 -> [w505 _]
                  frame False {
                    n83 = Wait on Notification(notifier=w505, timeout in ms (-1)=50) -> (notification=w503:T29, timed out?=w506:bool)  [unwired: 2 in, 2 out]
                    n84 = case shown="False" w506 {
                      tunnel: w509 -> [w513 _]
                      tunnel: w508 -> [w512 _]
                      tunnel: w507 -> [w511 _]
                      tunnel: w503 -> [w510 _]
                      frame False {
                        n85 = stacked-sequence {
                          seq-local: [w520 _ _ _ _ _] -> [_ w536 w539 w546 w562 _]
                          tunnel: w513 -> [w522 _ _ w554 w563 _]
                          tunnel: w512 -> [w518 _ _ _ _ _]
                          tunnel: w511 -> [w527 _ _ w548 _ _]
                          tunnel: w510 -> [_ _ _ _ _ w576]
                          frame #0 {
                            # "DISPLAY DATA"
                            n86 = Unbundle By Name(w518) -> ("ComError"=→"adam_nodata":bool, "Adam_Data"=w517:dbl[])
                            n87 = Unbundle By Name(w527) -> ("Mass"=w521:dbl)
                            n88 = Index Array(array=w517) -> (element=w515:dbl)  [unwired: 1 in]
                            n89 = Unbundle By Name(w522) -> ("PV"=w519:dbl, "wSP"=w524:dbl, "wOP"=w523:dbl)
                            n90 = call "_Data_in-range.vi"("data"=w515) -> ("data out"=w514:dbl)  [unwired: 3 in, 1 out]
                            "Sample Temperature" <- w514
                            n91 = Bundle("Mass"=w521, "PV"=w519, "data out"=w514) -> (w520:cluster{"Mass":dbl, "PV":dbl, "data out":dbl})  [unwired: 1 in]
                            n92 = Bundle By Name(cluster=T4 {"PV"=1800.0, "SP"=1600.0, "OP"=100.0} ("Eurotherm_3504"), "PV"=w519, "SP"=w524, "OP"=w523) -> (→"Eurotherm_3504":T4)
                            "Euro_Data_cluster" <- w522
                            "Balance_Data_cluster" <- w527
                            "Adam_Data_cluster" <- w518
                          }
                          frame #1 {
                            # "Display 2"
                            n93 = Number To Boolean Array(number="Adam_Out_FB") -> (Boolean array=w533:bool[])
                            n94 = Unbundle By Name(w536) -> ("Mass"=w535:dbl)
                            "Mass" <- w535
                            n95 = Index Array(array=w533, index #4=8 ("index")) -> (element #1=→"F1_Solenoid_On":bool, element #2=→"F2_Solenoid_On":bool, element #3=→"TGA_Gas_select" →"TGA_select_valve":bool, element #4=→"Adam_Out_Error":bool)  [unwired: 3 in]
                            n96 = Subtract(x=w535, y="Mass_offset") -> (x-y=→"Balance" →"Mass-Offset":dbl)
                            "Cluster" <- w536
                          }
                          frame #2 {
                            # "Update Chart every \n2nd call (1/sec)"
                            # "CHART - update every second point (1/sec)"
                            n97 = case shown="True" "chart" {
                              selector: "chart" -> [w543 w545]
                              tunnel: w539 -> [w544 _]
                              tunnel: [w543 w545] -> w541
                              frame False {
                                "Waveform Chart" <- w544
                              }
                              frame True {
                              }
                            }
                            n98 = Not(x=w541) -> (.not. x?=w540:bool)
                            n99 = local write "chart"(w540) -> ()
                          }
                          frame #3 {
                            # "DATA LOGGING"
                            n100 = Unbundle By Name(w548) -> ("Units"=→"Units":string)
                            n101 = Unbundle By Name(w554) -> ("Timestamp"=w553:dbl)
                            n102 = local read "Log File Path"() -> (w560:path)
                            n103 = local read "Logging"() -> (w559:bool)
                            n104 = local read "LogDivider"() -> (w558:i32)
                            n105 = Cluster To Array(cluster=w546) -> (array=w552:dbl[])
                            n106 = call "LogData.vi"("date/time"=w553, "Divisor"=w558, "Logging"=w559, "Data_cluster"=w546, "file path"=w560) -> ("Sample#"=→"Sample#":i32, "Elapsed Time (s)"=w555:i32)  [unwired: 5 in]
                            n107 = Not A Number/Path/Refnum?(number/path/refnum=w552) -> (NaN/Path/Refnum?=w551:bool[])
                            n108 = Index Array(array=w551) -> (element #1=→"balance_nodata":bool, element #2=→"eurotherm_nodata":bool)  [unwired: 2 in]
                            n109 = call "Seconds to hh-mm-ss.vi"("Elapsed Seconds"=w555) -> ("Elapsed Time (hh:mm:ss)"=→"Elapsed Time (hh:mm:ss)":string)
                          }
                          frame #4 {
                            # "Update Chart\n 1/s"
                            # "X-Y GRAPH"
                            n110 = local read "chart"() -> (w561:bool)
                            n111 = case shown="False" w561 {
                              tunnel: w563 -> [_ w571]
                              tunnel: w562 -> [_ w570]
                              frame False {
                              }
                              frame True {
                                n112 = Unbundle By Name(w571) -> ("Timestamp"=w568:dbl)
                                n113 = Cluster To Array(cluster=w570) -> (array=w565:dbl[])
                                n114 = local read "ClearGraph"() -> (w564:bool)
                                n115 = case shown="True" w564 {
                                frame False {
                                }
                                frame True {
                                n116 = local write "ClearGraph"(FALSE) -> ()
                                }
                                }
                                n117 = call "BuildXYGraph.vi"("ArraySizeLimit"="GraphSizeLimit", "Initialise"=w564, "DataArray"=w565, "date/time"=w568) -> ("XY Graph Array"=→"XY Graph":cluster{dbl[], dbl[]}[])  [unwired: 5 in]
                                n118 = case shown="\"Run\", Default" "Update Graph" {
                                tunnel: w568 -> [w573 _]
                                frame "Run", Default {
                                n119 = local read "ChrtWidth (s)"() -> (w574:i32)
                                n120 = Subtract(x=w573, y=w574) -> (x-y=w575:dbl)
                                n121 = property on="XY Graph" class="XYGraph (strict)"("XScale.Maximum"=w573, "XScale.Minimum"=w575) -> ()  [unwired: 2 in, 2 out]
                                }
                                frame "Pause" {
                                }
                                }
                              }
                            }
                          }
                          frame #5 {
                            # "Programmer"
                            "Prog read variables" <- w576
                          }
                        }
                      }
                      frame True {
                      }
                    }
                  }
                  frame True {
                  }
                }
              }
              frame True {
              }
            }
          }
          frame True {
          }
        }
        n122 = local read "stopping"() -> (w482:bool)
      }
      n123 = while "User Interface Events Loop" {
        tunnel: [w260] -> w148
        tunnel: w147 -> [w259]
        tunnel: w139 -> [w258]
        tunnel: w138 -> [w257]
        tunnel: w118 -> [w254]
        tunnel: [w254] -> w126
        tunnel: w119 -> [w255]
        stop <- w260 stop-if-true
        # "User Interface Events Loop"
        n124 = control-ref of="Gas Setpoints"() -> (w256:refnum<vi>)
        n125 = event shown="[15] \"Gas_Controls\": Value Change" {
          selector: _ -> [_ _ _ _ _ _ _ _ _ _ _ _ _ _ _ _ _ _ _ _ _ _ _]
          dyn-events: _ -> [_ _ _ _ _ _ _ _ _ _ _ _ _ _ _ _ _ _ _ _ _ _ _]
          timeout: _ -> [_ _ _ _ _ _ _ _ _ _ _ _ _ _ _ _ _ _ _ _ _ _ _]
          tunnel: [w262 w270 w280 _ _ _ _ _ _ _ _ _ _ _ _ _ _ _ _ _ _ _ _] -> w260
          tunnel: w259 -> [_ _ _ _ w296 _ w321 _ _ _ _ _ _ _ _ _ _ _ _ _ _ _ _]
          tunnel: w258 -> [_ _ _ _ _ _ _ _ _ _ _ w341 _ _ _ _ _ _ _ _ _ _ _]
          tunnel: w257 -> [_ _ _ _ _ _ _ _ _ _ _ _ _ w366 w368 _ _ _ _ _ _ _ _]
          tunnel: w256 -> [_ _ _ _ _ _ _ _ _ _ _ _ _ _ _ _ _ w405 w422 _ _ _ _]
          tunnel: w254 -> [_ _ _ _ _ _ _ _ _ _ _ _ _ _ _ w374 _ _ _ w429 _ _ _]
          tunnel: w255 -> [_ _ _ _ _ _ _ _ _ _ _ _ w364 _ _ _ _ _ _ _ _ _ _]
          event "stop": Value Change {
            n126 = event-data() -> ("NewVal"=w261:bool)  [unwired: 1 in]
            n127 = case shown="True" w261 {
              selector: w261 -> [w263 _]
              tunnel: [w263 w264] -> w262
              frame False {
              }
              frame True {
                # "Get confirmation"
                n128 = Two Button Dialog(message="Quit TGA Furnace\nData Logger Software.\n\nConfirm ?", 1:"No" ("F button name (\"Cancel\")"), 2:"Yes" ("T button name (\"OK\")")) -> (T button?=w264:bool)
              }
            }
          }
          event Panel Close? {
            n129 = event-data() -> ()  [unwired: 1 in, 1 out]
            n130 = local read "Logging"() -> (w268:bool)
            n131 = case shown="False" w268 {
              tunnel: [w274 w276] -> w270
              frame False {
                # "Get confirmation"
                n132 = Two Button Dialog(message="Quit TGA Furnace\nData Logger Software.\n\nConfirm ?", 1:"No" ("F button name (\"Cancel\")"), 2:"Yes" ("T button name (\"OK\")")) -> (T button?=w274:bool)
              }
              frame True {
                n133 = call <vilib>:"Beep.vi"() -> ()  [unwired: 12 in]
                n134 = Two Button Dialog(message="Warning:  Logging is active!\n\nIt is recommended that you stop logging first.\nIf you continue the log file will not be closed properly.\n", 2:"Ignore & Stop" ("T button name (\"OK\")")) -> (T button?=w276:bool)  [unwired: 1 in]
              }
            }
            n135 = event-data("Discard?"=TRUE) -> ()  [unwired: 1 in, 1 out]
          }
          event "stop": Mouse Up {
            n136 = event-data() -> ("CtlRef"=w279:refnum<vi>)  [unwired: 1 in]
            n137 = property class="Bool"(reference=w279) -> ("DisabledEnum"=w278:T27)  [unwired: 1 in, 2 out]
            n138 = Greater Than 0?(x=w278) -> (x > 0?=w281:bool)
            n139 = case shown="True" w281 {
              tunnel: [FALSE FALSE] -> w280
              frame False {
              }
              frame True {
                n140 = call <vilib>:"Beep.vi"() -> ()  [unwired: 12 in]
                n141 = One Button Dialog(message="QUIT is disabled.\n\nLogging must be \nstopped before quitting.") -> ()  [unwired: 1 in, 1 out]
              }
            }
          }
          event Value Change {
            n142 = event-data() -> ("NewVal"=w289:T6)  [unwired: 1 in]
            n143 = case shown="0, Default" w289 {
              tunnel: [60 300 600 1800 3600 7200] -> w286
              frame 0, Default {
              }
              frame 1 {
              }
              frame 2 {
              }
              frame 3 {
              }
              frame 4 {
              }
              frame 5 {
              }
            }
            "ChrtWidth (s)" <- w286
            n144 = Get Date/Time In Seconds() -> (seconds since 1Jan1904=w285:timestamp)
            n145 = To Double Precision Float(number=w285) -> (double precision float=w287:dbl)
            n146 = Subtract(x=w287, y=w286) -> (x-y=w288:dbl)
            n147 = property on="XY Graph" class="XYGraph (strict)"("X Scale.Range:Maximum"=w287, "X Scale.Range:Minimum"=w288) -> ()  [unwired: 2 in, 2 out]
          }
          event "StartLog_btn": Value Change {
            n148 = event-data() -> ("NewVal"=w297:bool)  [unwired: 1 in]
            n149 = case shown="True" w297 {
              tunnel: w296 -> [w299 _]
              frame True {
                n150 = call "StartLog.vi"("LogEndComment"="LogStartComment", "Data Directory Path"="Data directory path") -> ("error out"=w302:errorcluster, "Filename"=→"Filename":string, "Log File Path"=→"Log File Path":path)  [unwired: 5 in]
                n151 = case shown="No Error" w302 {
                  selector: w302 -> [_ w318]
                  tunnel: w299 -> [w304 _]
                  frame No Error {
                    n152 = stacked-sequence {
                      tunnel: w304 -> [w305 _ _]
                      frame #0 {
                        # "Wait for next data to synchronise\ntiming."
                        n153 = Wait on Notification(notifier=w305, timeout in ms (-1)=1000) -> ()  [unwired: 2 in, 4 out]
                      }
                      frame #1 {
                        "Logging" <- TRUE ("Logging")
                      }
                      frame #2 {
                        w308 = u8 2 ("Disabled")
                        n154 = property on="StartLog_btn" class="Bool"("Disabled"=w308) -> ()  [unwired: 2 in, 2 out]
                        n155 = property on="stop" class="Bool"("Disabled"=w308) -> ()  [unwired: 2 in, 2 out]
                        n156 = property on="Data directory path" class="Path"("Disabled"=w308) -> (error out=w309:errorcluster)  [unwired: 2 in, 1 out]
                        n157 = property on="StopLog_btn" class="Bool"("Disabled"=u8 0) -> ()  [unwired: 2 in, 2 out]
                        n158 = property on="offset_btn" class="Bool"(error in=w309, "DisabledEnum"=w308) -> ()  [unwired: 1 in, 2 out]
                      }
                    }
                  }
                  frame Error {
                    n159 = Unbundle By Name(w318) -> ("code"=w314:i32, "source"=w317:string)
                    n160 = Format Into String(format string="%d\n", initial string="ERROR:\n\n", w314) -> (resulting string=w311:string)  [unwired: 1 in, 1 out]
                    n161 = Concatenate Strings(w311, w317, "\n\n Couldn't open log file!\nTry again in 1 minute.") -> (w315:string)
                    n162 = One Button Dialog(message=w315) -> ()  [unwired: 1 in, 1 out]
                  }
                }
              }
              frame False {
              }
            }
          }
          event "StartLog_btn": Mouse Up {
            n163 = event-data() -> ("CtlRef"=w320:refnum<vi>)  [unwired: 1 in]
            n164 = property class="Bool"(reference=w320) -> ("DisabledEnum"=w319:T27)  [unwired: 1 in, 2 out]
            n165 = case shown="\"Disabled\", \"Disabled and Grayed Out\"" w319 {
              frame "Enabled", Default {
              }
              frame "Disabled", "Disabled and Grayed Out" {
                n166 = call <vilib>:"Beep.vi"() -> ()  [unwired: 12 in]
              }
            }
          }
          event "StopLog_btn": Value Change {
            n167 = event-data() -> ("NewVal"=w322:bool)  [unwired: 1 in]
            n168 = case shown="True" w322 {
              tunnel: w321 -> [w323 _]
              frame True {
                n169 = stacked-sequence {
                  tunnel: w323 -> [_ w326 _ _]
                  frame #0 {
                    # "Set logging OFF and disable stop button"
                    n170 = property on="StopLog_btn" class="Bool"("Disabled"=u8 2) -> ()  [unwired: 2 in, 2 out]
                    n171 = local write "Logging"(FALSE) -> ()
                  }
                  frame #1 {
                    # "Wait until next data available to ensure logging has stopped"
                    n172 = Wait on Notification(notifier=w326, timeout in ms (-1)=400) -> ()  [unwired: 2 in, 4 out]
                  }
                  frame #2 {
                    # "Get postscript comments"
                    n173 = local read "Log File Path"() -> (w329:path)
                    n174 = call "StopLog.vi"("GetComment"="LogEndComment", "Log File Path"=w329) -> ()  [unwired: 7 in, 1 out]
                  }
                  frame #3 {
                    w330 = u8 0 ("Disabled")
                    # "Re-enable StartLog, Quit and Log File Data Directory control."
                    n175 = property on="StartLog_btn" class="Bool"("Disabled"=w330) -> ()  [unwired: 2 in, 2 out]
                    n176 = property on="stop" class="Bool"("Disabled"=w330) -> ()  [unwired: 2 in, 2 out]
                    n177 = property on="Data directory path" class="Path"("Disabled"=w330) -> ()  [unwired: 2 in, 2 out]
                    n178 = property on="offset_btn" class="Bool"("DisabledEnum"=w330) -> ()  [unwired: 2 in, 2 out]
                  }
                }
              }
              frame False {
              }
            }
          }
          event "StopLog_btn": Mouse Up {
            n179 = event-data() -> ("CtlRef"=w332:refnum<vi>)  [unwired: 1 in]
            n180 = property class="Bool"(reference=w332) -> ("DisabledEnum"=w331:T27)  [unwired: 1 in, 2 out]
            n181 = case shown="\"Disabled\", \"Disabled and Grayed Out\"" w331 {
              frame "Enabled", Default {
              }
              frame "Disabled", "Disabled and Grayed Out" {
                # "Button disabled - beep"
                n182 = call <vilib>:"Beep.vi"() -> ()  [unwired: 12 in]
              }
            }
          }
          event Value Change {
            n183 = event-data() -> ("NewVal"=→"LogDivider":T1)  [unwired: 1 in]
          }
          event "clear_graph": Value Change {
            n184 = event-data() -> ()  [unwired: 1 in, 1 out]
            n185 = case shown="True" "clear_graph" {
              frame False {
              }
              frame True {
                n186 = Two Button Dialog(message="This will clear all traces from the graph.\nContinue ?") -> (T button?=→"ClearGraph":bool)  [unwired: 2 in]
              }
            }
          }
          event "offset_btn": Value Change {
            n187 = event-data() -> ()  [unwired: 1 in, 1 out]
            n188 = local read "Mass"() -> (w337:dbl)
            n189 = Not A Number/Path/Refnum?(number/path/refnum=w337) -> (NaN/Path/Refnum?=w338:bool)
            n190 = case shown="False" w338 {
              tunnel: w337 -> [w339 _]
              frame False {
                n191 = local write "Mass_offset"(w339) -> ()
              }
              frame True {
                n192 = call <vilib>:"Beep.vi"() -> ()  [unwired: 12 in]
              }
            }
          }
          event "Temp_SP_btn": Mouse Up {
            n193 = event-data() -> ("Mods.Double Click"=w340:bool)  [unwired: 1 in]
            n194 = case shown="True" w340 {
              tunnel: w341 -> [_ w344]
              frame False {
              }
              frame True {
                n195 = local read "Eurotherm_3504"() -> (w343:T4)
                n196 = Unbundle By Name(w343) -> ("SP"=w342:dbl)
                n197 = call "Euro_SP_Adjust_dialog.vi"("Temp_SP"=w342, "EuroCmd_queue"=w344) -> ()  [unwired: 10 in]
              }
            }
          }
          event "Euro_cmd_Write Cluster": Value Change {
            n198 = event-data() -> ()  [unwired: 1 in, 6 out]
            n199 = local read "Euro_cmd_Write Cluster"() -> (w345:T17)
            n200 = Unbundle By Name(w345) -> ("Writeable_Registers"=w361:T16, "Value"=w360:bool, "Writeable_Registers 2"=w359:T16, "Value 2"=w358:bool, "Writeable_Registers 3"=w357:T16, "Value 3"=w356:bool, "Writeable_Registers 4"=w355:T16, "d/min"=w354:u16, "Writeable_Registers 5"=w353:T16, "deg"=w352:u16, "Writeable_Registers 6"=w351:T16, "(m)"=w350:u16, "Writeable_Registers 7"=w349:T16, "d/min"=w348:u16, "Writeable_Registers 8"=w347:T16, "deg"=w346:u16)
            n201 = Bundle By Name(cluster=T28 {"Register"=5446, "Value"=FALSE, "Value 2"=FALSE, "Register 2"=5445, "Value 3"=FALSE, "Register 3"=5412, "Value 4"=0.0, "Register 4"=0, "Value 5"=0.0, "Register 5"=5382, "Value 6"=0.0, "Register 6"=5412, "Value 7"=0.0, "Register 7"=5445, "Value 8"=0.0, "Register 8"=5446, "Value 9"=0.0, "Register 9"=470} ("EuroCmd_cluster_2"), "Register"=w361, "Value"=w360, "Register 2"=w359, "Value 2"=w358, "Register 3"=w357, "Value 3"=w356, "Register 4"=w355, "Value 4"=w354, "Register 5"=w353, "Value 5"=w352, "Register 6"=w351, "Value 6"=w350, "Register 7"=w349, "Value 7"=w348, "Register 8"=w347, "Value 8"=w346) -> (w363:T28)
            n202 = Enqueue Element(queue=w364, element=w363) -> ()  [unwired: 2 in, 3 out]
          }
          event "Tare_Balance_btn": Value Change {
            n203 = event-data() -> ()  [unwired: 1 in, 1 out]
            n204 = Enqueue Element(queue=w366, element=T30 {"cmd"=enum."Tare", "Value"=0}) -> ()  [unwired: 2 in, 3 out]
          }
          event "Zero_Balance_btn": Value Change {
            n205 = event-data() -> ()  [unwired: 1 in, 1 out]
            n206 = Enqueue Element(queue=w368, element=T30 {"cmd"=enum."Zero", "Value"=0}) -> ()  [unwired: 2 in, 3 out]
          }
          event "Gas_Controls": Value Change {
            n207 = event-data() -> ("NewVal.H2 On"=w372:bool, "NewVal.CO On"=w371:bool, "NewVal.CO2 On"=w370:bool, "NewVal.N2 On"=w369:bool)  [unwired: 1 in]
            n208 = Compound Arithmetic op=OR(w372, w371, w370, w369) -> (w373:bool)
            n209 = case shown="True" w373 {
              tunnel: w374 -> [w376 w389]
              frame False {
                n210 = local write "Gas_Controls"(T8 {"N2 On"=TRUE, "H2 On"=FALSE, "CO On"=FALSE, "CO2 On"=FALSE} ("Gas_Controls")) -> ()
                n211 = Build Array(FALSE ("element"), FALSE ("element"), TRUE) -> (w380:bool[])
                n212 = Boolean Array To Number(Boolean array=w380) -> (number=w379:u32)
                n213 = To Unsigned Byte Integer(number=w379) -> (unsigned 8bit integer=w377:u8)
                n214 = Send Notification(notification=w377, notifier=w376) -> ()  [unwired: 1 in, 2 out]
                "cancel_purge" <- FALSE
              }
              frame True {
                w388 = FALSE  # RDI-2 Sol
                w384 = TRUE  # Shared sol + TGA select sol
                n215 = Build Array(w384, w388, w384) -> (w387:bool[])
                n216 = Boolean Array To Number(Boolean array=w387) -> (number=w386:u32)
                n217 = To Unsigned Byte Integer(number=w386) -> (unsigned 8bit integer=w385:u8)
                n218 = Send Notification(notification=w385, notifier=w389) -> ()  [unwired: 1 in, 2 out]
              }
            }
          }
          event "Gas Setpoints": Value Change {
            # "Make N2 = the balance of 100%"
            n219 = event-data() -> ("NewVal"=w395:T9)  [unwired: 1 in]
            n220 = Unbundle By Name(w395) -> ("F1 CO (%)"=w396:dbl, "F1 CO2 (%)"=w397:dbl, "F1 H2 (%)"=w398:dbl)
            n221 = Compound Arithmetic op=ADD(w396, w397, w398) -> (w400:dbl)
            n222 = Subtract(x=100.0 ("y"), y=w400) -> (x-y=w401:dbl)
            n223 = Bundle By Name(cluster=w395, "F1 N2 (%)"=w401) -> (w394:T9)
            n224 = Not Equal?(x="Gas_SPs_Loaded", y=w394) -> (x != y?=w392:T35)
            n225 = local write "Gas Setpoints"(w394) -> ()
            n226 = Cluster To Array(cluster=w392) -> (array=w391:bool[])
            n227 = Or Array Elements(Boolean array=w391) -> (logical OR=→"Gasfile_changed":bool)
          }
          event "gasfile_open_btn": Value Change {
            n228 = event-data() -> ()  [unwired: 1 in, 1 out]
            n229 = local read "Gas_Filename"() -> (w407:string)
            n230 = call "_Load-Save_Gas_File.vi"("Mode (Load)"=enum16{"Load", "Save", "SaveAs"}."Load", "Gas_Setpoints_ref"=w405, "Gas_Filename"=w407) -> ("Loaded"=w403:bool, "Gas_SPs_out"=w402:T9, "Gas_Filepath"=w404:path)  [unwired: 5 in, 1 out]
            n231 = case shown="True" w403 {
              tunnel: w404 -> [_ w410]
              tunnel: w402 -> [_ w409]
              frame False {
              }
              frame True {
                n232 = local write "Gas_SPs_Loaded"(w409) -> ()
                n233 = Strip Path(path=w410) -> (name=w412:string)  [unwired: 1 out]
                n234 = Match Pattern(string=w412, regular expression="\\.") -> (before substring=→"Gas_Filename":string)  [unwired: 1 in, 3 out]
                n235 = local write "Gasfile_changed"(FALSE ("Gasfile_changed")) -> ()
              }
            }
          }
          event "gasfile_save_btn", "gasfile_saveas_btn": Value Change {
            n236 = event-data() -> ()  [unwired: 1 in, 1 out]
            n237 = local read "Gas_Filename"() -> (w421:string)
            n238 = Select(t=enum16{"Load", "Save", "SaveAs"}."Save" ("Mode (Load)"), s="gasfile_save_btn", f=enum16{"Load", "Save", "SaveAs"}."SaveAs" ("Mode (Load)")) -> (s? t:f=w418:enum16{"Load", "Save", "SaveAs"})
            n239 = call "_Load-Save_Gas_File.vi"("Mode (Load)"=w418, "Gas_Setpoints_ref"=w422, "Gas_Filename"=w421) -> ("Saved"=w420:bool, "Gas_SPs_out"=w414:T9, "Gas_Filepath"=w419:path)  [unwired: 5 in, 1 out]
            n240 = case shown="True" w420 {
              tunnel: w419 -> [_ w428]
              tunnel: w414 -> [_ w424]
              frame False {
              }
              frame True {
                n241 = Strip Path(path=w428) -> (name=w426:string)  [unwired: 1 out]
                n242 = local write "Gas_SPs_Loaded"(w424) -> ()
                n243 = Match Pattern(string=w426, regular expression="\\.") -> (before substring=w425:string)  [unwired: 1 in, 3 out]
                n244 = local write "Gasfile_changed"(FALSE ("Gasfile_changed")) -> ()
                n245 = local write "Gas_Filename"(w425) -> ()
              }
            }
          }
          event "N2_Alarm_2": Value Change {
            # "Set/reset by reference in 'Detect N2 Alarm' subVI"
            n246 = event-data() -> ("NewVal"=w430:bool)  [unwired: 1 in]
            n247 = case shown="True" w430 {
              tunnel: w429 -> [_ w432]
              frame False {
              }
              frame True {
                # "N2 low flow alarm - turn gas off"
                n248 = local write "Gas_Controls"(T8 {"N2 On"=FALSE, "H2 On"=FALSE, "CO On"=FALSE, "CO2 On"=FALSE} ("Gas_Controls")) -> ()
                n249 = Send Notification(notification=u8 0, notifier=w432) -> ()  [unwired: 1 in, 2 out]
              }
            }
          }
          event Value Change {
            n250 = event-data() -> ("NewVal"=w434:T11, "OldVal"=w438:T11)  [unwired: 1 in]
            "Purge_state_indicator" <- w434
            n251 = Not Equal?(x=w434, y=w438) -> (x != y?=w437:bool)
            n252 = Index Array(array=u32[] [13816530, 16776960, 65535, 16776960, 16749459, 16776960, 9228031], index=w434) -> (element=w436:u32)
            n253 = property on="Purge_state_indicator" class="Enum (strict)"("RingText.BGColor"=w436) -> ()  [unwired: 2 in, 2 out]
            n254 = case shown="False" w437 {
              tunnel: w434 -> [_ w440]
              frame False {
              }
              frame True {
                n255 = case shown="\"StartReduction\", \"Reduction\"" w440 {
                  tunnel: [T8 {"N2 On"=FALSE, "H2 On"=FALSE, "CO On"=FALSE, "CO2 On"=FALSE} ("Gas_Controls") T8 {"N2 On"=TRUE, "H2 On"=FALSE, "CO On"=FALSE, "CO2 On"=FALSE} ("Gas_Controls") w446 w455] -> w439
                  tunnel: [FALSE TRUE TRUE TRUE] -> w441
                  frame "Ready", Default {
                  }
                  frame "StartPrePurge", "PrePurge" {
                  }
                  frame "StartReduction", "Reduction" {
                    n256 = local read "Gas Setpoints"() -> (w451:T9)
                    n257 = Unbundle(w451) -> ("F1 H2 (%)"=w450:dbl, "F1 CO (%)"=w448:dbl, "F1 CO2 (%)"=w449:dbl)  [unwired: 2 out]
                    n258 = Build Array(1.0 ("element"), w450, w448, w449) -> (w452:dbl[])
                    n259 = Array To Cluster(array=w452) -> (cluster=w453:T36)
                    n260 = Greater Than 0?(x=w453) -> (x > 0?=w446:T37)
                  }
                  frame "StartPostPurge", "PostPurge" {
                    n261 = local read "Purge Setpoints"() -> (w456:T12)
                    n262 = Greater Than 0?(x=w456) -> (x > 0?=w455:T38)
                  }
                }
                n263 = property on="Gas_Controls" class="Clust (strict)"("Val(Sgnl)"=w439) -> ()  [unwired: 2 in, 2 out]
                n264 = property on="Remaining" class="DigNum (strict)"("Visible"=w441) -> ()  [unwired: 2 in, 2 out]
              }
            }
            n265 = call <vilib>:"Beep.vi"() -> ()  [unwired: 12 in]
          }
          event "PrePurge Time", "Gas_Times.Reduction Time", "Gas_Times.Purge Time": Mouse Up {
            n266 = event-data() -> ("CtlRef"=w459:refnum<vi>, "Coords"=w460:T39, "Mods.Double Click"=w461:bool)  [unwired: 1 in]
            n267 = property class="VI"() -> ("Front Panel.WinBounds"=w458:T40)  [unwired: 2 in, 2 out]
            n268 = case shown="True" w461 {
              tunnel: w460 -> [_ w463]
              tunnel: w459 -> [_ w462]
              tunnel: w458 -> [_ w467]
              frame False {
              }
              frame True {
                n269 = Unbundle By Name(w463) -> ("Horizontal"=w470:i32, "Vertical"=w468:i32)
                n270 = Unbundle By Name(w467) -> ("Left"=w471:i16, "Top"=w469:i16)
                n271 = Add(x=w468, y=w469) -> (x+y=w465:i32)
                n272 = Add(x=w470, y=w471) -> (x+y=w466:i32)
                n273 = Bundle By Name(cluster=w463, "Horizontal"=w466, "Vertical"=w465) -> (w464:T39)
                n274 = call "_Adjust_Timer_SP_xRef.vi"("Coords"=w464, "CtlRef"=w462) -> ()  [unwired: 10 in]
              }
            }
          }
          event "Purge Setpoints": Value Change {
            n275 = event-data() -> ("CtlRef"=w474:refnum<vi>, "NewVal"=w473:T12)  [unwired: 1 in]
            n276 = Unbundle By Name(w473) -> ("F1 CO (%)"=w475:dbl, "F1 CO2 (%)"=w476:dbl, "F1 H2 (%)"=w477:dbl)
            n277 = Compound Arithmetic op=ADD(w475, w476, w477) -> (w479:dbl)
            n278 = Subtract(x=100.0 ("y"), y=w479) -> (x-y=w480:dbl)
            n279 = Bundle By Name(cluster=w473, "F1 N2 (%)"=w480) -> (w472:T12)
            n280 = property class="Clust (strict)"(reference=w474, "Value"=w472) -> ()  [unwired: 1 in, 2 out]
          }
        }
      }
      "stopping" <- w148
      n281 = call "Initialise TGA MFCs.vi"("number of retries (5)"=w125, "MFC Device IDs in"=w127, "VISA resource name"=w128) -> ("ValveStatus"=w130:u8[], "Init Errors"=→"MFC Init. Error":bool[], "SVs"=w131:dbl[], "VISA Refnum out"=w135:refnum<visa-resource-name>, "MFC Device IDs out"=w132:T26[])  [unwired: 4 in]
      n282 = call "Balance_IO_Loop.vi"("Balance_cmd_queue"=w138, "Balance_Notifier"=w147, "VISA name"=w144) -> ("reference out"=w122:refnum<vi>)  [unwired: 8 in]
      n283 = call "Adam-ID_Input_Loop.vi"("Adam_In_Notifier"=w145, "Adam_ID_cluster"=w143) -> ("reference out"=w124:refnum<vi>)  [unwired: 9 in]
      n284 = call "Eurotherm_IO_Loop.vi"("EuroCmd_queue 2"=w119, "Eurotherm_Notifier 2"=w120, "EuroCmd_queue"=w139, "Eurotherm_Notifier"=w146, "Address (1)"=w141, "VISA name"=w142) -> ("reference out"=w123:refnum<vi>)  [unwired: 5 in]
      n285 = while "MFCs IO Loop" {
        shift-left: w130 -> [w190]
        shift-right: [w165] -> _
        shift-left: _ -> [w192]
        shift-right: [w193] -> _
        tunnel: [w196] -> w134
        shift-left: w131 -> [w197]
        shift-right: [w155] -> _
        tunnel: w132 -> [w199]
        tunnel: w135 -> [w198]
        tunnel: w118 -> [w152]
        tunnel: [w151] -> w117
        stop <- w181 stop-if-true
        w156 = 600 ("Numeric")
        # "Event generated\nvia this refnum."
        # "MFCs IO Loop"
        n286 = control-ref of="cancel_purge"() -> (w167:refnum<vi>)
        n287 = call "_Purge_state_machine.vi"("cancel_purge_ref"=w167, "stop_btn"="stop_red_btn", "start_btn"="start_red_btn", "PrePurge Time"=w156, "Purge_Times"="Gas_Times") -> ("Changed"=w166:bool, "Remaining"=→"Remaining":i32, "State"=w161:T11)  [unwired: 2 in]
        n288 = Cluster To Array(cluster="Gas_Controls") -> (array=w180:bool[])
        n289 = call "TGAGas_SPs_to_Flow_SPs.vi"("Purge_Flow"="Purge Flow", "State"=w161, "Purge Setpoints"="Purge Setpoints", "Gas Setpoints"="Gas Setpoints") -> ("Flow_SP_Array"=w184:dbl[])  [unwired: 7 in]
        n290 = for {
          tunnel: w184 -> [w203] mode=indexing
          tunnel: w180 -> [w207] mode=indexing
          tunnel: w199 -> [w214] mode=indexing
          tunnel: w198 -> [w215]
          tunnel: [w213] -> w196
          tunnel: [w212] -> w194 mode=indexing
          tunnel: [w201] -> w155 mode=indexing
          tunnel: w197 -> [w208] mode=indexing
          tunnel: [w211] -> w185 mode=indexing
          tunnel: [w202] -> w179 mode=indexing
          tunnel: [w209] -> w165 mode=indexing
          tunnel: w190 -> [w210] mode=indexing
          tunnel: "Flow_error%" -> [w206]
          tunnel: [w205] -> w160 mode=indexing
          i -> [w217]
          n291 = Increment(x=w217) -> (x+1=→"MFC Scan":i32)
          n292 = call "_MFC_read-write.vi"("VISA Refnum"=w215, "MFC Device ID"=w214, "Flow SP"=w203, "Prev Flow PV"=w208, "Valve Status"=w210, "Gas On"=w207, "number of retries (5)"=1) -> ("MFC Update"=w212:bool, "VISA Refnum out"=w213:refnum<visa-resource-name>, "SV Out"=w202:dbl, "Flow PV"=w201:dbl, "Valve Status out"=w209:u8, "MFC Error"=w211:bool)  [unwired: 3 in]
          n293 = call "_Detect_low_flow.vi"("Error (%)"=w206, "Gas_On"=w207, "PV"=w201, "Read SP"=w202) -> ("Flow_state"=w205:enum16{"Off", "Ok", "Low"})  [unwired: 5 in]
        }
        "MFC Errors" <- w185
        "Read Setpoints" <- w179
        "Actual Flows (l/min)" <- w155
        "MFC Update" <- w194
        n294 = case shown="True" w166 {
          tunnel: w161 -> [_ w200]
          frame False {
          }
          frame True {
            n295 = property on="Purge_State" class="Enum (strict)"("Val(Sgnl)"=w200) -> ()  [unwired: 2 in, 2 out]
          }
        }
        n296 = Add Array Elements(numeric array=w179) -> (sum=w189:dbl)
        n297 = Tick Count (ms)() -> (millisecond timer value=w193:u32)
        n298 = call "Door lock output.vi"("Test flow"="test flow", "Array"=w155, "Notifier in"=w152) -> (0:→"lock door", "Notifier out"=w151:refnum<notifier>)  [unwired: 7 in]
        n299 = Add Array Elements(numeric array=w155) -> (sum=→"Actual Flow (l/min)":dbl)
        n300 = Or Array Elements(Boolean array=w185) -> (logical OR=→"MFC com error":bool)
        n301 = Equal To 0?(x=w189) -> (x = 0?=→"All Gas Off":bool)
        n302 = Equal?(x=w165, y=u8 2) -> (x = y?=→"Sol Valve States":bool[])
        n303 = Subtract(x=w193, y=w192) -> (x-y=→"MFC Loop (ms)":u32)
        n304 = Array To Cluster(array=w160) -> (cluster=→"Flow_status_cluster":T41)
        n305 = Array To Cluster(array=w155) -> (cluster=→"Gas_Flows" →"Gas_Flows 2":T36)
        n306 = control-ref of="N2_Alarm_2"() -> (w162:refnum<vi>)
        n307 = Or(x="reset_btn2", y="reset_alarm_btn") -> (x .or. y?=w174:bool)
        n308 = call "_Detect_N2_Alarm.vi"("N2_Alarm_ref"=w162, "reset_alarm_btn"=w174, "AlarmDelay"="AlarmDelay", "Flow_State_array"=w160) -> ("N2_Alarm"=w158:bool, "N2_flow_state"=→"N2_Flow_state":enum16{"Off", "Ok", "Low"})  [unwired: 6 in]
        "N2_Alarm" <- w158
        n309 = local read "stopping"() -> (w181:bool)
        n310 = property on="reset_alarm_btn" class="Bool"("Visible"=w158) -> ()  [unwired: 2 in, 2 out]
        "PrePurge Time" <- w156
      }
      n311 = call "Adam-ID_output_Loop.vi"("Adam_Out_Notifier"=w117, "OP_feedback_ref"=w136, "Adam_ID_cluster"=w137) -> ("reference out"=w121:refnum<vi>)  [unwired: 8 in]
      n312 = flat-sequence {
        tunnel: [w218] -> w140
        tunnel: w140 -> [w230]
        frame #0 {
          n313 = while "Display About page for 8 seconds" {
            tunnel: [w226] -> w218
            i -> [w223]
            stop <- w225 stop-if-true
            n314 = local read "Tab Control"() -> (w227:T2)
            n315 = Subtract(x=100 ("y"), y=w223) -> (x-y=w221:i32)
            "Slide" <- w221
            n316 = Equal To 0?(x=w221) -> (x = 0?=w220:bool)
            n317 = local read "stopping"() -> (w224:bool)
            n318 = Not Equal?(x=w227, y=T19."About" ("Tab Control")) -> (x != y?=w226:bool)
            n319 = Wait (ms)(milliseconds to wait=u32 80) -> ()  [unwired: 1 out]
            n320 = Compound Arithmetic op=OR(w226, w220, w224) -> (w225:bool)
          }
        }
        frame #1 {
          w229 = FALSE ("Visible")
          n321 = case shown="True" w230 {
            frame False {
              n322 = local write "Tab Control"(T19."Display" ("Tab Control")) -> ()
            }
            frame True {
            }
          }
          n323 = property on="Slide" class="Slide (strict)"("Visible"=w229) -> ()  [unwired: 2 in, 2 out]
          "Config_Load_Error" <- w229
        }
      }
      n324 = stacked-sequence "Save Config Data before quitting" {
        seq-local: [w233 _] -> [_ w253]
        tunnel: w129 -> [w239 _]
        tunnel: [_ w251] -> w150
        tunnel: w148 -> [_ _]
        frame #0 {
          n325 = local read "Data directory path"() -> (w240:path)
          n326 = local read "LogStartComment"() -> (w237:bool)
          n327 = local read "LogEndComment"() -> (w236:bool)
          n328 = local read "GraphSizeLimit"() -> (w234:i32)
          n329 = local read "GraphWidth"() -> (w235:T6)
          n330 = local read "LogInterval"() -> (w238:T1)
          n331 = Bundle By Name(cluster=w239, "Data directory path"=w240, "LogInterval"=w238, "LogStartComment"=w237, "LogEndComment"=w236, "GraphWidth"=w235, "GraphSizeLimit"=w234) -> (w233:T21)
        }
        frame #1 {
          n332 = local read "Purge Setpoints"() -> (w244:T12)
          n333 = local read "Gas_Times"() -> (w243:cluster{"Reduction Time":i32, "Purge Time":i32})
          n334 = local read "Gas_Filename"() -> (w248:string)
          n335 = local read "Gas Setpoints"() -> (w247:T9)
          n336 = local read "Flow_error%"() -> (w245:dbl)
          n337 = local read "Purge Flow"() -> (w249:dbl)
          n338 = local read "AlarmDelay"() -> (w246:dbl)
          n339 = Unbundle(w243) -> ("Reduction Time"=w242:i32, "Purge Time"=w241:i32)
          n340 = Bundle By Name(cluster=w253, "TGA Gas File"=w248, "Gas_SPs"=w247, "AlarmDelay"=w246, "Flow_error%"=w245, "Purge Flow"=w249, "Gas_Times.Reduction Time"=w242, "Gas_Times.Purge Time"=w241, "Purge Setpoints"=w244) -> (w250:T21)
          n341 = call "Load-Save Configuration.vi"("Save (F: Load)"=TRUE, "Config Cluster"=w250) -> ("Error"=w251:bool)  [unwired: 6 in, 1 out]
        }
      }
      n342 = Release Notifier(notifier=w126) -> ()  [unwired: 2 in, 3 out]
      n343 = for {
        tunnel: string[] ["BalanceLoop", "AdamLoop", "EurothermLoop"] -> [w232] mode=indexing
        tunnel: w148 -> [_]
        n344 = call <vilib>:"Stop Timed Structure.vi"("name"=w232) -> ()  [unwired: 10 in, 1 out]
      }
      n345 = VISA Close(VISA resource name=w134) -> ()  [unwired: 1 in, 1 out]
    }
  }
  n346 = stacked-sequence "Quit" {
    tunnel: w14 -> [_ _]
    tunnel: w6 -> [w580 _]
    tunnel: w5 -> [w581 _]
    tunnel: w4 -> [w579 _]
    tunnel: w3 -> [w578 _]
    frame #0 {
      n347 = Build Array(w579, w578, w580, w581) -> (w577:refnum<vi>[])
      n348 = for {
        tunnel: w577 -> [w582] mode=indexing
        n349 = invoke class="VI" method="FP.Close"(reference=w582) -> ()  [unwired: 2 in, 3 out]
      }
    }
    frame #1 {
      n350 = invoke class="VI" method="FP.Close"() -> ()  [unwired: 3 in, 3 out]
    }
  }
